vi "GUI control.vi"() -> ()   [LabVIEW 2018]
doc: "This example performs a serial port write and a serial port read. The parameters set for the serial port must match the parameters of the connected instrument or device. The VISA Configure Serial Port VI sets the configuration parameters. The front panel displays the controls used to configure the basic parameters, such as baud rate, data bits, and parity. The VI passes the VISA resource name to other VIs that perform operations on that VISA resource. The VISA Write function sends a command to the serial device and the VISA Read function returns data based on the command. The VISA Close function then closes the reference to the serial device. It is important to close the reference; otherwise, further communication through that port might not be possible."
uses:
  Program Files/National Instruments/LabVIEW 2018/examples/Instrument IO/Serial/support/Serial - Settings.ctl
  <vilib>/Instr/_visa.llb/VISA Configure Serial Port (Instr).vi
  <vilib>/Utility/file.llb/Write Delimited Spreadsheet (string).vi
panel:
  in  "file path 1D":path
  in  "file path static":path
  out "Magnetic field z [µT]":dbl
  out "Magnetic field y [µT]":dbl
  out "Magnetic field x [µT]":dbl
  out "Magnetic field strength [µT]":dbl
  in  "Direction field sweep":string(combo)
  in  "Minimum value B [µT]":dbl
  in  "Maximum value B [µT]":dbl
  in  "START":bool
  in  "Number of steps":dbl
  out "Current has stabilized":bool
  in  "Next iteration 2":bool
  in  "Starting step":dbl
  out "Current has stabilized":bool
  out "Current has stabilized":bool
  in  "Next iteration":bool
  in  "file path 3D":path
  in  "Start":bool
  out "Start time 2":timestamp
  out "Angle \"phi\"":dbl
  out "Current iteration":i32
  in  "Number of steps":dbl
  in  "Angle theta [degrees]":dbl
  in  "Magnetic field strength [µT]":dbl
  in  "Octant":string(combo)
  in  "Sweep plane & fixed axis":string(combo)
  in  "OFF":bool
  in  "OK Button":bool
  in  "Magnetic field strength z [µT]":dbl
  in  "Magnetic field strength y [µT]":dbl
  in  "Magnetic field strength x [µT]":dbl
  in  "Static or field sweep?":string(combo)
  in  "Serial Settings":T1={"baud rate"=9600, "data bits"=8, "parity"=enum."None", "stop bits"=10, "flow control"=0} {"flow control" items=["None"=0, "XON/XOFF"=1, "RTS/CTS"=2, "DTR/DSR"=4]; "stop bits" items=["1.0"=10, "1.5"=15, "2.0"=20]; "data bits" min=5 max=8 step=1; "baud rate" items=["75"=75, "110"=110, "134"=134, "150"=150, "300"=300, "600"=600, "1200"=1200, "1800"=1800, "2400"=2400, "4800"=4800, "7200"=7200, "9600"=9600, "14400"=14400, "19200"=19200, "28800"=28800, "38400"=38400, "56000"=56000, "57600"=57600, "115200"=115200, "128000"=128000, "230400"=230400]}
  in  "VISA resource name":refnum<visa-resource-name>="COM1"
  # "Static field"
  # "1D magnitude sweep"
  # "Settings"
  # "3D field sweep"
  # "About the 3D field sweep"
  # "A onstant-magnitude, fixed-tilt, azimuthal sweep of a 3D vector is performed.\nThe mag,netic field vector is angled away from a fixed axis by a certain angle \"phi\". It then makes a circular motion around that fixed axis, eventually tracing out a full cone.\nYou choose a plane of variation ( x–y, x–z, or y–z) and hold one direction constant (e.g., z).  The sweep is performed clockwise, as seen from the origin."
  # "File paths must be a csv comma delimited excell file!"
  # "How to connect the cables"
  # "Current state"
  # "Current state"
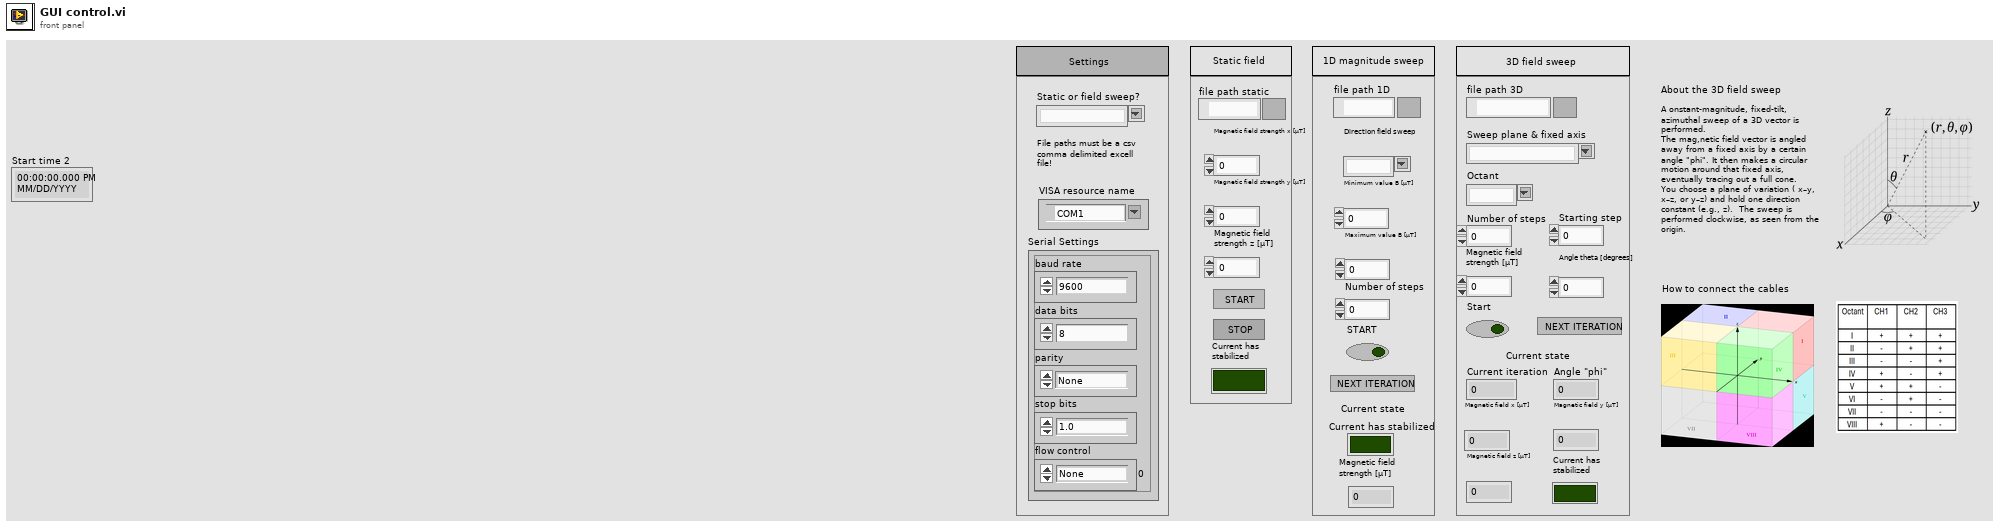
[diagram p1: front panel]
types:
  T1 = typedef "Serial - Settings.ctl" = cluster{"baud rate":u32, "data bits":u16, "parity":enum16{"None", "Odd", "Even", "Mark", "Space"}, "stop bits":u16, "flow control":u16}
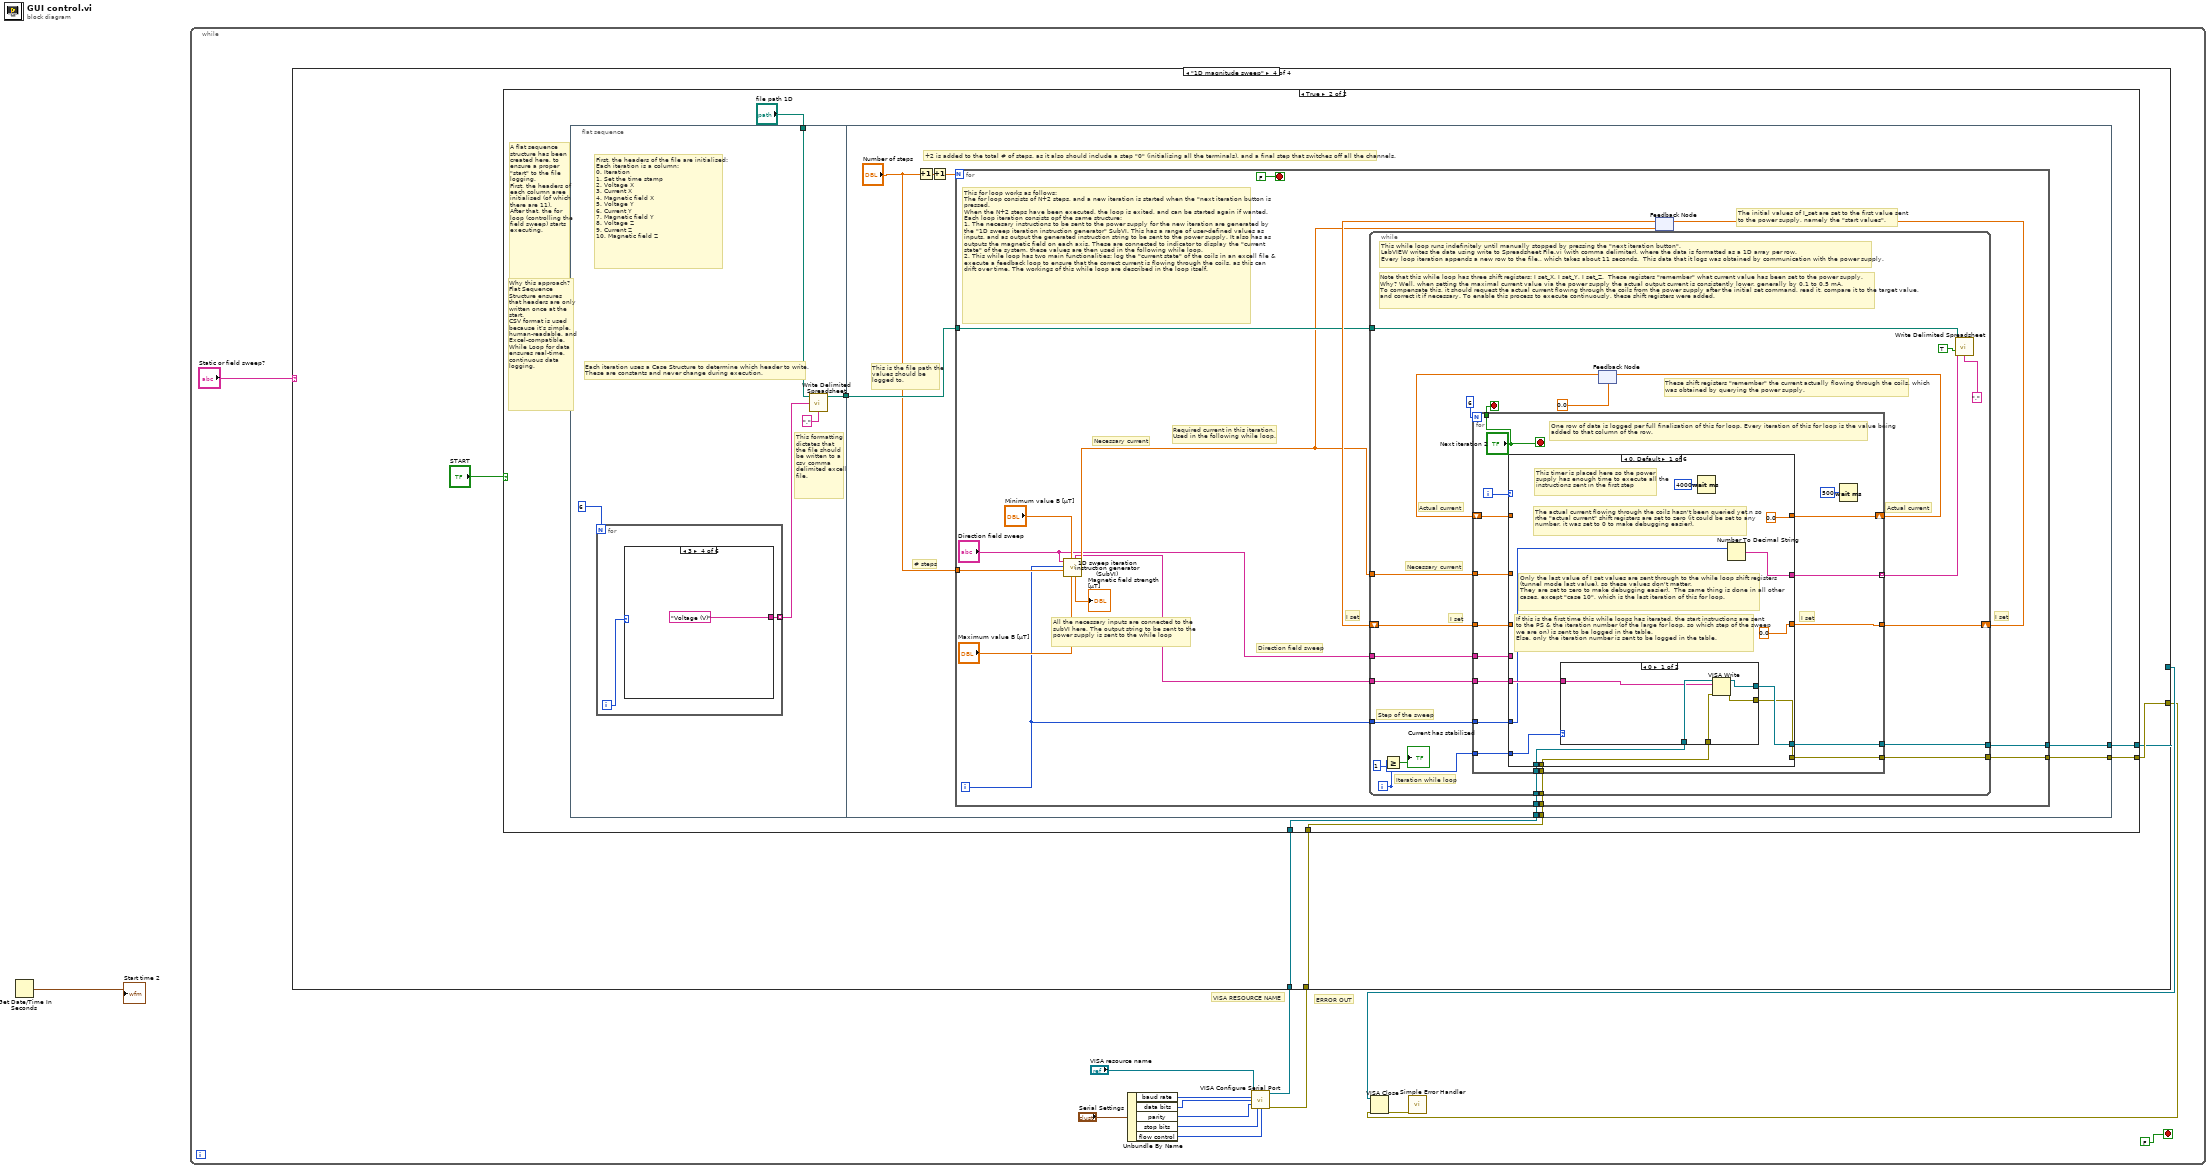
[diagram p0: block diagram]
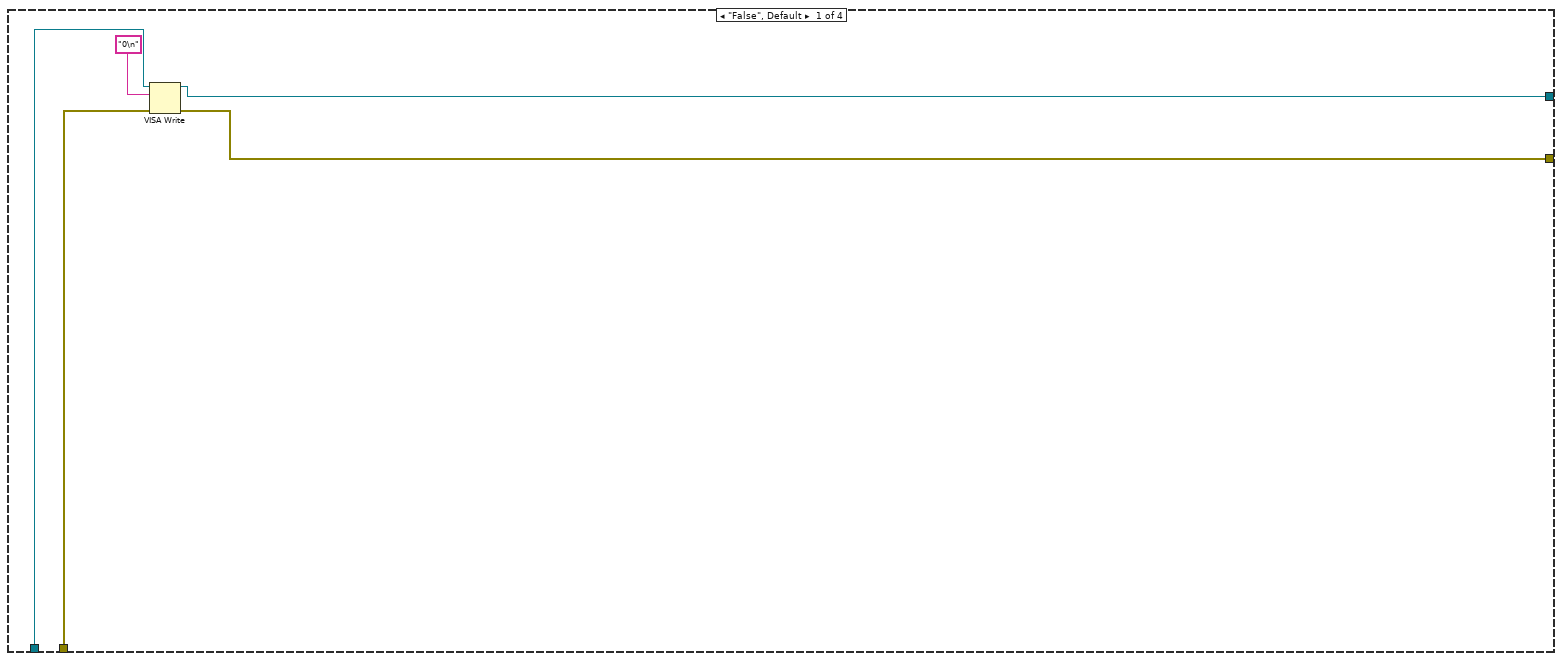
[diagram p2: hidden frame]
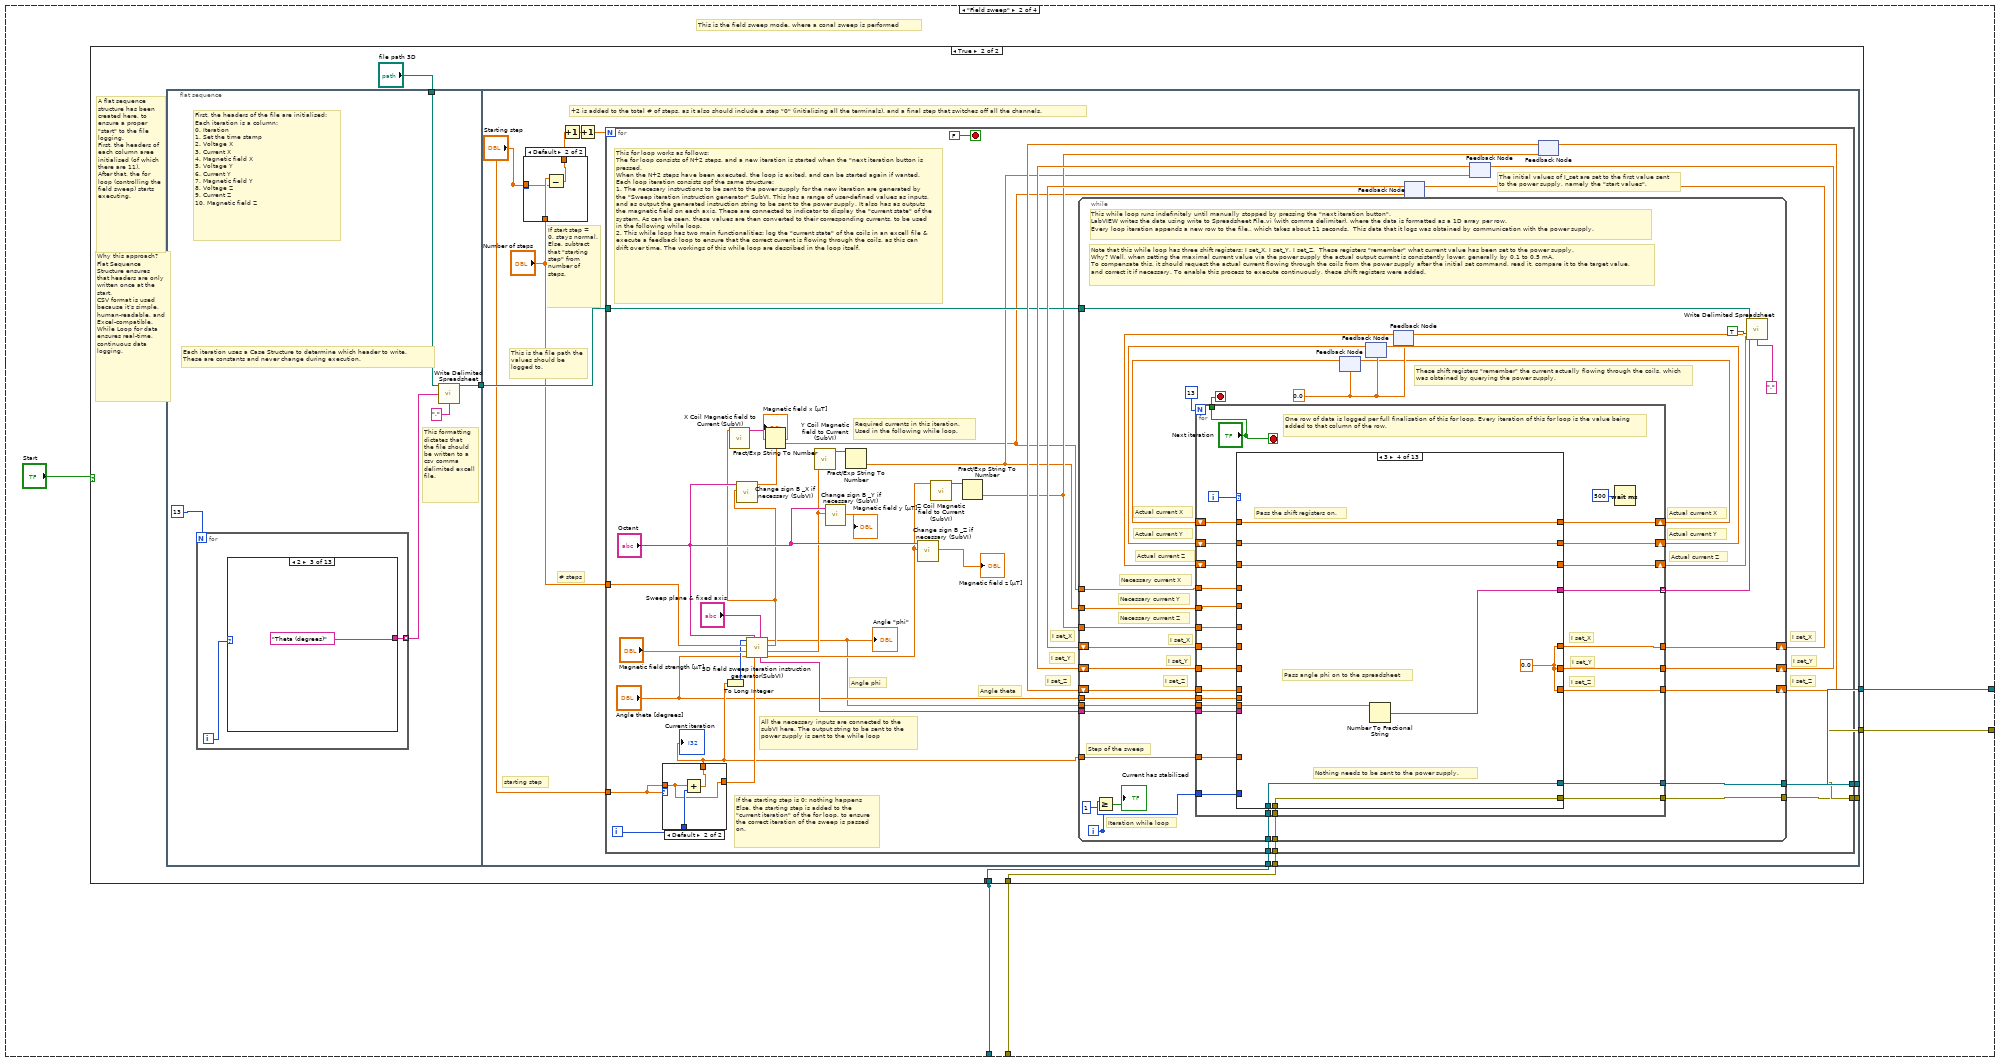
[diagram p3: hidden frame]
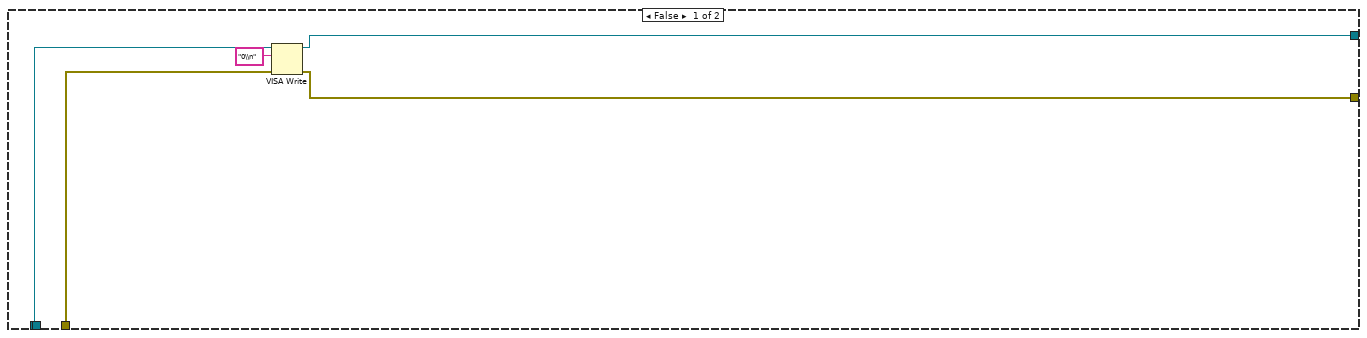
[diagram p4: hidden frame]
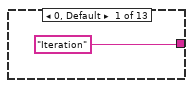
[diagram p5: hidden frame]
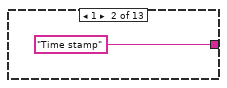
[diagram p6: hidden frame]
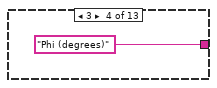
[diagram p7: hidden frame]
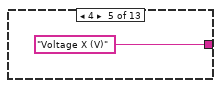
[diagram p8: hidden frame]
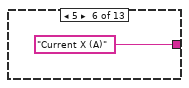
[diagram p9: hidden frame]
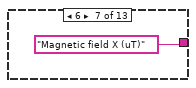
[diagram p10: hidden frame]
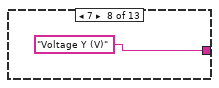
[diagram p11: hidden frame]
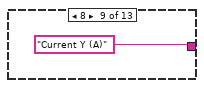
[diagram p12: hidden frame]
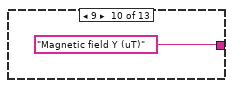
[diagram p13: hidden frame]
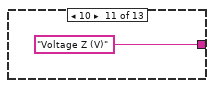
[diagram p14: hidden frame]
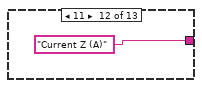
[diagram p15: hidden frame]
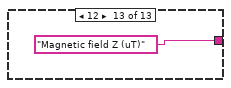
[diagram p16: hidden frame]
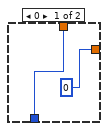
[diagram p18: hidden frame]
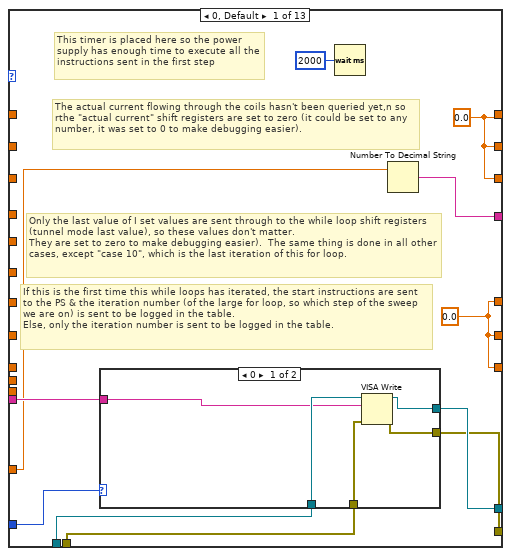
[diagram p19: hidden frame]
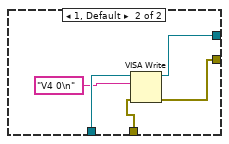
[diagram p20: hidden frame]
diagram:
  n1 = Get Date/Time In Seconds() -> (seconds since 1Jan1904=→"Start time 2":timestamp)
  n2 = while {
    stop <- FALSE stop-if-true
    # "VISA RESOURCE NAME"
    # "ERROR OUT"
    n3 = Unbundle By Name("Serial Settings") -> ("baud rate"=w12:u32, "data bits"=w2:u16, "parity"=w11:enum16{"None", "Odd", "Even", "Mark", "Space"}, "stop bits"=w10:u16, "flow control"=w9:u16)
    n4 = call-poly "VISA Configure Serial Port"("VISA resource name"="VISA resource name", "baud rate (9600)"=w12, "data bits (8)"=w2, "parity (0:none)"=w11, "stop bits (10: 1 bit)"=w10, "flow control (0:none)"=w9) -> ("VISA resource name out"=w3:refnum<visa-resource-name>, "error out"=w8:errorcluster)  [unwired: 3 in, 5 out]
    n5 = case shown="\"1D magnitude sweep\"" "Static or field sweep?" {
      tunnel: [w16 w24 w444 w813] -> w6
      tunnel: w3 -> [w18 w22 w441 w815]
      tunnel: w8 -> [w19 w23 w445 w814]
      tunnel: [w17 w25 w443 w812] -> w7
      frame "False", Default {
        n6 = VISA Write(VISA resource name=w18, write buffer="0\n", error in (no error)=w19) -> (VISA resource name out=w17:refnum<visa-resource-name>, error out=w16:errorcluster)  [unwired: 1 out]
      }
      frame "Field sweep" {
        # "This is the field sweep mode, where a conal sweep is performed"
        n7 = case shown="True" "Start" {
          tunnel: [w30 w34] -> w25
          tunnel: [w29 w33] -> w24
          tunnel: w22 -> [w27 w36]
          tunnel: w23 -> [w28 w35]
          tunnel: w22 -> [_ _]
          frame False {
            n8 = VISA Write(VISA resource name=w27, write buffer="0\\n", error in (no error)=w28) -> (VISA resource name out=w30:refnum<visa-resource-name>, error out=w29:errorcluster)  [unwired: 1 out]
          }
          frame True {
            # "Why this approach?\nFlat Sequence Structure ensures that headers are only written once at the start.\nCSV format is used because it’s simple, human-readable, and Excel-compatible.\nWhile Loop for data ensures real-time, continuous data logging."
            # "A flat sequence structure has been created here, to ensure a proper \"start\" to the file logging. \nFirst, the headers of each column aree initialised (of which there are 11). \nAfter that, the for loop (controlling the field sweep) starts executing."
            n9 = flat-sequence {
              tunnel: "file path 3D" -> [w38]
              tunnel: [w37] -> w32
              tunnel: w36 -> [w64]
              tunnel: w35 -> [w63]
              tunnel: [w62] -> w34
              tunnel: [w61] -> w33
              tunnel: w32 -> [w60]
              frame #0 {
                # "Each iteration uses a Case Structure to determine which header to write.\nThese are constants and never change during execution."
                # "This formatting dictates that the file should be written to a csv comma delimited excell file."
                # "First, the headers of the file are initialised:\nEach iteration is a column:\n0. Iteration\n1. Set the time stamp\n2. Voltage X\n3. Current X\n4. Magnetic field X\n5. Voltage Y\n6. Current Y\n7. Magnetic field Y\n8. Voltage Z\n9. Current Z\n10. Magnetic field Z"
                n10 = for {
                  N: 13 -> [_]
                  tunnel: [w42] -> w40 mode=indexing
                  i -> [w43]
                  n11 = case shown="2" w43 {
                    tunnel: ["Iteration" "Time stamp" "Theta (degrees)" "Phi (degrees)" "Voltage X (V)" "Current X (A)" "Magnetic field X (uT)" "Voltage Y (V)" "Current Y (A)" "Magnetic field Y (uT)" "Voltage Z (V)" "Current Z (A)" "Magnetic field Z (uT)"] -> w42
                    frame 0, Default {
                    }
                    frame 1 {
                    }
                    frame 2 {
                    }
                    frame 3 {
                    }
                    frame 4 {
                    }
                    frame 5 {
                    }
                    frame 6 {
                    }
                    frame 7 {
                    }
                    frame 8 {
                    }
                    frame 9 {
                    }
                    frame 10 {
                    }
                    frame 11 {
                    }
                    frame 12 {
                    }
                  }
                }
                n12 = call-poly <vilib>:"Write Delimited Spreadsheet.vi"("file path (dialog if empty)"=w38, "1D data"=w40, "delimiter (\\t)"="," ("delimiter (\\t)")) -> ("new file path (Not A Path if cancelled)"=w37:path)  [unwired: 11 in, 1 out]
              }
              frame #1 {
                # "starting step"
                # "# steps"
                # "If start step = 0, stays normal.\nElse, subtract that \"starting step\" from number of steps."
                # "This is the file path the values should be logged to."
                # "+2 is added to the total # of steps, as it also should include a step \"0\" (initialising all the terminals), and a final step that switches off all the channels."
                n13 = case shown="Default" "Starting step" {
                  tunnel: "Number of steps" -> [w67 w70]
                  tunnel: [w67 w69] -> w58
                  tunnel: "Starting step" -> [_ w68]
                  frame 0 {
                  }
                  frame Default {
                    n14 = Subtract(x=w70, y=w68) -> (x-y=w69:dbl)
                  }
                }
                n15 = Increment(x=w58) -> (x+1=w66:dbl)
                n16 = Increment(x=w66) -> (x+1=w65:dbl)
                n17 = for {
                  N: w65 -> [_]
                  tunnel: "Number of steps" -> [w101]
                  tunnel: w64 -> [w92]
                  tunnel: w63 -> [w91]
                  tunnel: [w90] -> w62
                  tunnel: [w89] -> w61
                  tunnel: w60 -> [w88]
                  tunnel: "Starting step" -> [w80]
                  i -> [w81]
                  stop <- FALSE stop-if-true
                  # "Angle phi"
                  # "Angle theta"
                  # "If the starting step is 0: nothing happens\nElse, the starting step is added to the \"current iteration\" of the for loop, to ensure the correct iteration of the sweep is passed on."
                  # "The initial values of I_set are set to the first value sent to the power supply, namely the \"start values\"."
                  # "All the necessary inputs are connected to the subVI here. The output string to be sent to the power supply is sent to the while loop"
                  # "This for loop works as follows: \nThe for loop consists of N+2 steps, and a new iteration is started when the \"next iteration button is pressed.\nWhen the N+2 steps have been executed, the loop is exited, and can be started again if wanted.\nEach loop iteration consists opf the same structure:\n1. The necesary instructions to be sent to the power supply for the new iteration are generated by the \"Sweep iteration instruction generator\" SubVI. This has a range of user-defined values as inputs, and as output the generated instruction string to be sent to the power supply. It also has as outputs the magnetic field on each axis. These are connected to indicator to display the \"current state\" of the system. As can be seen, these values are then converted to their corresponding currents, to be used in the following while loop.\n2. This while loop has two main functionalities: log the \"current state\" of the coils in an excell file & execute a feedback loop to ensure that the correct current is flowing through the coils, as this can drift over time. The workings of this while loop are described in the loop itself."
                  # "I set_Z"
                  # "I set_Y"
                  # "I set_Y"
                  # "I set_Z"
                  # "I set_X"
                  # "I set_X"
                  # "Required currents in this iteration. \nUsed in the following while loop."
                  n18 = case shown="Default" w80 {
                    tunnel: w81 -> [w108 w111]
                    tunnel: [w108 w110] -> w75
                    tunnel: w80 -> [_ w109]
                    tunnel: [0 ("y") w109] -> w79
                    frame 0 {
                    }
                    frame Default {
                      n19 = Add(x=w109, y=w111) -> (x+y=w110:dbl)
                    }
                  }
                  "Current iteration" <- w75
                  n20 = To Long Integer(number=w75) -> (32bit integer=w74:i32)
                  n21 = call "3D field sweep iteration instruction generator(SubVI).vi"("Sweep plane & fixed axis"="Sweep plane & fixed axis", "Sweep starts later"=w79, "Octant"="Octant", "Angle theta [degrees]"="Angle theta [degrees]", "Magnetic field strength [µT]"="Magnetic field strength [µT]", "Number of steps"=w101, "Current iteration"=w74) -> ("Magnetic field z [µT]"=w76:dbl, "Magnetic field y [µT]"=w77:dbl, "Magnetic field x [µT]"=w78:dbl, "Azimuthal angle \"phi\""=w71:dbl, "Output string instruction"=w93:string)
                  "Angle \"phi\"" <- w71
                  n22 = call "X Coil Magnetic field to Current (SubVI).vi"("Magnetic field [µT]"=w78) -> ("Current X"=w103:string)  [unwired: 10 in]
                  n23 = call "Change sign B _X if necessary (SubVI).vi"("Magnetic field x [µT] in"=w78, "Octant"="Octant") -> ("Magnetic field x [µT] out"=→"Magnetic field x [µT]":dbl)  [unwired: 9 in]
                  n24 = Fract/Exp String To Number(string=w103) -> (number=w82:dbl)  [unwired: 3 in, 1 out]
                  n25 = call "Y Coil Magnetic field to Current (SubVI).vi"("Magnetic field [µT]"=w77) -> ("Current Y"=w104:string)  [unwired: 10 in]
                  n26 = call "Change sign B _Y if necessary (SubVI).vi"("Magnetic field y [µT]  in"=w77, "Octant"="Octant") -> ("Magnetic field y [µT]  out"=→"Magnetic field y [µT]":dbl)  [unwired: 9 in]
                  n27 = Fract/Exp String To Number(string=w104) -> (number=w86:dbl)  [unwired: 3 in, 1 out]
                  n28 = call "Change sign B _Z if necessary (SubVI).vi"("Magnetic field z [µT] in"=w76, "Octant"="Octant") -> ("Magnetic field z [µT] out"=→"Magnetic field z [µT]":dbl)  [unwired: 9 in]
                  n29 = call "Z Coil Magnetic field to Current (SubVI).vi"("Magnetic field [µT]"=w76) -> ("Current Z"=w105:string)  [unwired: 10 in]
                  n30 = Fract/Exp String To Number(string=w105) -> (number=w87:dbl)  [unwired: 3 in, 1 out]
                  n31 = feedback #1(w82) -> (w99:dbl)
                  n32 = feedback #2(w86) -> (w96:dbl)
                  n33 = feedback #3(w87) -> (w94:dbl)
                  n34 = while {
                    tunnel: w88 -> [w141]
                    tunnel: w92 -> [w138]
                    tunnel: w91 -> [w137]
                    tunnel: [w136] -> w89
                    tunnel: [w135] -> w90
                    tunnel: w75 -> [w128]
                    shift-right: [w127] -> w98
                    shift-left: w99 -> [w126]
                    tunnel: w93 -> [w125]
                    shift-right: [w124] -> w97
                    shift-left: w96 -> [w122]
                    shift-right: [w123] -> w95
                    shift-left: w94 -> [w121]
                    tunnel: w82 -> [w120]
                    tunnel: w86 -> [w119]
                    tunnel: w87 -> [w118]
                    tunnel: "Angle theta [degrees]" -> [w113]
                    tunnel: w71 -> [w112]
                    i -> [w117]
                    stop <- w114 stop-if-true
                    w130 = 0.0
                    # "These shift registers \"remember\" the current actually flowing through the coils, which was obtained by querying the power supply."
                    # "Note that this while loop has three shift registers: I set_X, I set_Y, I set_Z.  These registers \"remember\" what current value has been set to the power supply. \nWhy? Well, when setting the maximal current value via the power supply the actual output current is consistently lower, generally by 0.1 to 0.5 mA.\nTo compensate this, it should request the actual current flowing through the coils from the power supply after the initial set command, read it, compare it to the target value, and correct it if necessary. To enable this process to execute continuously, these shift registers were added."
                    # "This while loop runs indefinitely until manually stopped by pressing the \"next iteration button\". \nLabVIEW writes the data using write to Spreadsheet File.vi (with comma delimiter), where the data is formatted as a 1D array per row.\nEvery loop iteration appends a new row to the file,, which takes about 11 seconds.  This data that it logs was obtained by communication with the power supply."
                    # "Necessary current Z"
                    # "Necessary current Y"
                    # "Necessary current X"
                    # "I set_Z"
                    # "I set_Y"
                    # "Iteration while loop"
                    # "Step of the sweep"
                    # "I set_X"
                    # "Actual current Z"
                    # "Actual current Y"
                    # "Actual current X"
                    # "Actual current Z"
                    # "Actual current Y"
                    # "Actual current X"
                    n35 = Greater Or Equal?(x=w117, y=1) -> (x >= y?=→"Current has stabilized":bool)
                    n36 = feedback #4(w130) -> (w143:dbl)
                    n37 = feedback #5(w130) -> (w133:dbl)
                    n38 = feedback #6(w130) -> (w131:dbl)
                    n39 = for {
                      N: 13 -> [_]
                      tunnel: [w170] -> w142 mode=indexing
                      shift-right: [w165] -> w129
                      shift-left: w143 -> [w172]
                      tunnel: w138 -> [w169]
                      tunnel: w137 -> [w168]
                      tunnel: [w167] -> w136
                      tunnel: [w166] -> w135
                      shift-right: [w162] -> w134
                      shift-left: w133 -> [w164]
                      shift-right: [w161] -> w132
                      shift-left: w131 -> [w163]
                      tunnel: w117 -> [w160]
                      tunnel: w128 -> [w159]
                      tunnel: w126 -> [w158]
                      tunnel: [w157] -> w127
                      tunnel: w125 -> [w156]
                      tunnel: [w155] -> w124
                      tunnel: [w154] -> w123
                      tunnel: w122 -> [w153]
                      tunnel: w121 -> [w152]
                      tunnel: w120 -> [w151]
                      tunnel: w119 -> [w150]
                      tunnel: w118 -> [w149]
                      tunnel: ["Next iteration"] -> w114
                      tunnel: w113 -> [w146]
                      tunnel: w112 -> [w145]
                      i -> [w171]
                      stop <- "Next iteration" stop-if-true
                      # "One row of data is logged per full finalisation of this for loop. Every iteration of this for loop is the value being added to that column of the row."
                      # "I set_Y"
                      # "I set_Z"
                      # "I set_X"
                      n40 = case shown="3" w171 {
                        tunnel: [w177 w200 w209 w213 w220 w247 w269 w279 w298 w321 w333 w356 w393] -> w170
                        tunnel: w169 -> [w180 w199 w204 w212 w235 w256 w271 w281 w305 w325 w335 w360 w386]
                        tunnel: w168 -> [w181 w198 w203 w211 w234 w257 w270 w280 w306 w326 w334 w359 w385]
                        tunnel: [w183 w199 w204 w212 w233 w259 w271 w275 w303 w325 w332 w358 w388] -> w166
                        tunnel: [w182 w198 w203 w211 w232 w258 w270 w274 w302 w326 w331 w357 w387] -> w167
                        tunnel: [w179 w197 w208 w217 w239 w248 w272 w278 w300 w324 w330 w355 w392] -> w165
                        tunnel: w172 -> [_ w197 w208 w217 w239 _ w272 w278 w300 w324 w330 w355 w392]
                        tunnel: w164 -> [_ w196 w207 w216 w223 w245 w268 w277 _ w322 w329 w354 w384]
                        tunnel: w163 -> [_ w195 w206 w215 w222 w244 w267 w276 w299 w323 w328 _ w380]
                        tunnel: [w179 w196 w207 w216 w223 w245 w268 w277 w301 w322 w329 w354 w384] -> w162
                        tunnel: [w179 w195 w206 w215 w222 w244 w267 w276 w299 w323 w328 w353 w380] -> w161
                        tunnel: w160 -> [w178 _ _ _ _ _ _ _ _ _ _ _ w375]
                        tunnel: w159 -> [w174 _ _ _ _ _ _ _ _ _ _ _ _]
                        tunnel: [w175 w194 w205 w218 w219 w243 w266 w273 w297 w320 w327 w352 w389] -> w157
                        tunnel: w158 -> [_ _ _ _ _ _ _ _ _ _ _ _ w391]
                        tunnel: w156 -> [w176 _ _ _ _ _ _ _ _ _ _ _ _]
                        tunnel: [w175 w194 w205 w218 w219 w243 w266 w273 w297 w320 w327 w352 w381] -> w155
                        tunnel: [w175 w194 w205 w218 w219 w243 w266 w273 w297 w320 w327 w352 w377] -> w154
                        tunnel: w153 -> [_ _ _ _ _ _ _ _ _ _ _ _ w383]
                        tunnel: w152 -> [_ _ _ _ _ _ _ _ _ _ _ _ w378]
                        tunnel: w151 -> [_ _ _ _ _ _ _ _ _ _ _ _ w390]
                        tunnel: w150 -> [_ _ _ _ _ _ _ _ _ _ _ _ w382]
                        tunnel: w149 -> [_ _ _ _ _ _ _ _ _ _ _ _ w379]
                        tunnel: w146 -> [_ _ w210 _ _ _ _ _ _ _ _ _ _]
                        tunnel: w145 -> [_ _ _ w214 _ _ _ _ _ _ _ _ _]
                        frame 0, Default {
                          w175 = 0.0
                          w179 = 0.0
                          # "This timer is placed here so the power supply has enough time to execute all the instructions sent in the first step"
                          # "Only the last value of I set values are sent through to the while loop shift registers (tunnel mode last value), so these values don't matter. \nThey are set to zero to make debugging easier).  The same thing is done in all other cases, except \"case 10\", which is the last iteration of this for loop."
                          # "The actual current flowing through the coils hasn't been queried yet,n so rthe \"actual current\" shift registers are set to zero (it could be set to any number, it was set to 0 to make debugging easier)."
                          # "If this is the first time this while loops has iterated, the start instructions are sent to the PS & the iteration number (of the large for loop, so which step of the sweep we are on) is sent to be logged in the table.\nElse, only the iteration number is sent to be logged in the table."
                          n41 = case shown="0" w178 {
                            tunnel: [w188 w193] -> w183
                            tunnel: [w187 w192] -> w182
                            tunnel: w181 -> [w186 w191]
                            tunnel: w180 -> [w185 w190]
                            tunnel: w176 -> [w184 _]
                            frame 0 {
                              n42 = VISA Write(VISA resource name=w185, write buffer=w184, error in (no error)=w186) -> (VISA resource name out=w188:refnum<visa-resource-name>, error out=w187:errorcluster)  [unwired: 1 out]
                            }
                            frame 1, Default {
                              n43 = VISA Write(VISA resource name=w190, write buffer="V4 0\n", error in (no error)=w191) -> (VISA resource name out=w193:refnum<visa-resource-name>, error out=w192:errorcluster)  [unwired: 1 out]
                            }
                          }
                          n44 = Wait (ms)(milliseconds to wait=u32 2000) -> ()  [unwired: 1 out]
                          n45 = Number To Decimal String(number=w174) -> (decimal integer string=w177:string)  [unwired: 1 in]
                        }
                        frame 1 {
                          w194 = 0.0
                          # "Nothing needs to be sent to the power supply."
                          # "Pass the shift registers on."
                          # "only send the time, not the date"
                          # "Send the time stamp to be logged"
                          n46 = Get Date/Time In Seconds() -> (seconds since 1Jan1904=w202:timestamp)
                          n47 = Format Date/Time String(time format string (%c)="%H:%M:%S", seconds (now)=w202) -> (date/time string=w200:string)  [unwired: 1 in]
                        }
                        frame 2 {
                          w205 = 0.0
                          # "Nothing needs to be sent to the power supply."
                          # "Pass the shift registers on."
                          # "Pass angle theta to the spreadsheet"
                          n48 = Number To Fractional String(number=w210) -> (F-format string=w209:string)  [unwired: 3 in]
                        }
                        frame 3 {
                          w218 = 0.0
                          # "Nothing needs to be sent to the power supply."
                          # "Pass angle phi on to the spreadsheet"
                          # "Pass the shift registers on."
                          n49 = Number To Fractional String(number=w214) -> (F-format string=w213:string)  [unwired: 3 in]
                        }
                        frame 4 {
                          w219 = 0.0
                          # "Pass the shift registers on."
                          # "The answer back from the PS is in the form x V. This V needs to be removed, otherwise the table formats wrong."
                          # "Request voltage CH1 & write it to the file"
                          n50 = call "Request voltage CH1 (SubVI).vi"() -> ("Request voltage CH1 / X"=w225:string)  [unwired: 11 in]
                          n51 = VISA Write(VISA resource name=w235, write buffer=w225, error in (no error)=w234) -> (VISA resource name out=w238:refnum<visa-resource-name>, error out=w237:errorcluster)  [unwired: 1 out]
                          n52 = flat-sequence {
                            tunnel: w237 -> [w240]
                            tunnel: w238 -> [w241]
                            tunnel: [w241] -> w231
                            tunnel: u32 500 ("delay before read (ms) static") -> [w242]
                            tunnel: [w240] -> w230
                            frame #0 {
                              n53 = Wait (ms)(milliseconds to wait=w242) -> ()  [unwired: 1 out]
                            }
                          }
                          n54 = property class="Instr"(reference=w231, error in=w230) -> (reference out=w229:refnum<visa-resource-name>, error out=w228:errorcluster, "Serial Settings:Number of Bytes at Serial Port"=w227:u32)
                          n55 = VISA Read(VISA resource name=w229, byte count=w227, error in (no error)=w228) -> (VISA resource name out=w233:refnum<visa-resource-name>, read buffer=w224:string, error out=w232:errorcluster)  [unwired: 1 out]
                          n56 = Scan From String(format string="%fV", input string=w224) -> (output 1=w221:dbl)  [unwired: 3 in, 3 out]
                          n57 = Number To Fractional String(number=w221) -> (F-format string=w220:string)  [unwired: 3 in]
                        }
                        frame 5 {
                          w243 = 0.0
                          # "Pass the shift registers on."
                          # "The answer back from the PS is in the form x A. This A needs to be removed, otherwise the table formats wrong."
                          # "Request current CH1; write it to the file; put it on the current X shift register"
                          n58 = call "Request current CH1(SubVI).vi"() -> ("Request current CH1 / X"=w249:string)  [unwired: 11 in]
                          n59 = VISA Write(VISA resource name=w256, write buffer=w249, error in (no error)=w257) -> (VISA resource name out=w262:refnum<visa-resource-name>, error out=w261:errorcluster)  [unwired: 1 out]
                          n60 = flat-sequence {
                            tunnel: w261 -> [w263]
                            tunnel: w262 -> [w264]
                            tunnel: [w264] -> w254
                            tunnel: u32 500 ("delay before read (ms) static") -> [w265]
                            tunnel: [w263] -> w253
                            frame #0 {
                              n61 = Wait (ms)(milliseconds to wait=w265) -> ()  [unwired: 1 out]
                            }
                          }
                          n62 = property class="Instr"(reference=w254, error in=w253) -> (reference out=w252:refnum<visa-resource-name>, error out=w250:errorcluster, "Serial Settings:Number of Bytes at Serial Port"=w251:u32)
                          n63 = VISA Read(VISA resource name=w252, byte count=w251, error in (no error)=w250) -> (VISA resource name out=w259:refnum<visa-resource-name>, read buffer=w255:string, error out=w258:errorcluster)  [unwired: 1 out]
                          n64 = Scan From String(format string="%fA", input string=w255) -> (output 1=w248:dbl)  [unwired: 3 in, 3 out]
                          n65 = Number To Fractional String(number=w248) -> (F-format string=w247:string)  [unwired: 3 in]
                        }
                        frame 6 {
                          w266 = 0.0
                          # "Pass the shift registers on."
                          # "Send magnetic field X to log file"
                          n66 = call "X Coil Current to Magnetic field (SubVI).vi"("Current X"=w272) -> ("Magnetic field X [µT]"=w269:string)  [unwired: 10 in]
                        }
                        frame 7 {
                          w273 = 0.0
                          # "Pass the shift registers on."
                          # "The answer back from the PS is in the form x V. This V needs to be removed, otherwise the table formats wrong."
                          # "Request voltage CH2 & write it to the file"
                          n67 = call "Request voltage CH2 (SubVI).vi"() -> ("Request voltage CH2 / Y"=w282:string)  [unwired: 11 in]
                          n68 = VISA Write(VISA resource name=w281, write buffer=w282, error in (no error)=w280) -> (VISA resource name out=w293:refnum<visa-resource-name>, error out=w292:errorcluster)  [unwired: 1 out]
                          n69 = flat-sequence {
                            tunnel: w292 -> [w294]
                            tunnel: w293 -> [w295]
                            tunnel: [w295] -> w290
                            tunnel: u32 500 ("delay before read (ms) static") -> [w296]
                            tunnel: [w294] -> w289
                            frame #0 {
                              n70 = Wait (ms)(milliseconds to wait=w296) -> ()  [unwired: 1 out]
                            }
                          }
                          n71 = property class="Instr"(reference=w290, error in=w289) -> (reference out=w288:refnum<visa-resource-name>, error out=w287:errorcluster, "Serial Settings:Number of Bytes at Serial Port"=w286:u32)
                          n72 = VISA Read(VISA resource name=w288, byte count=w286, error in (no error)=w287) -> (VISA resource name out=w275:refnum<visa-resource-name>, read buffer=w284:string, error out=w274:errorcluster)  [unwired: 1 out]
                          n73 = Scan From String(format string="%fV", input string=w284) -> (output 1=w283:dbl)  [unwired: 3 in, 3 out]
                          n74 = Number To Fractional String(number=w283) -> (F-format string=w279:string)  [unwired: 3 in]
                        }
                        frame 8 {
                          w297 = 0.0
                          # "Pass the shift registers on."
                          # "The answer back from the PS is in the form x A. This A needs to be removed, otherwise the table formats wrong."
                          # "Request current CH2; write it to the file; put it on the current Y shift register"
                          n75 = call "Request current CH2 (SubVI).vi"() -> ("Request current CH2 / Y"=w304:string)  [unwired: 11 in]
                          n76 = VISA Write(VISA resource name=w305, write buffer=w304, error in (no error)=w306) -> (VISA resource name out=w316:refnum<visa-resource-name>, error out=w315:errorcluster)  [unwired: 1 out]
                          n77 = flat-sequence {
                            tunnel: w315 -> [w317]
                            tunnel: w316 -> [w318]
                            tunnel: [w318] -> w312
                            tunnel: u32 500 ("delay before read (ms) static") -> [w319]
                            tunnel: [w317] -> w311
                            frame #0 {
                              n78 = Wait (ms)(milliseconds to wait=w319) -> ()  [unwired: 1 out]
                            }
                          }
                          n79 = property class="Instr"(reference=w312, error in=w311) -> (reference out=w310:refnum<visa-resource-name>, error out=w308:errorcluster, "Serial Settings:Number of Bytes at Serial Port"=w309:u32)
                          n80 = VISA Read(VISA resource name=w310, byte count=w309, error in (no error)=w308) -> (VISA resource name out=w303:refnum<visa-resource-name>, read buffer=w313:string, error out=w302:errorcluster)  [unwired: 1 out]
                          n81 = Scan From String(format string="%fA", input string=w313) -> (output 1=w301:dbl)  [unwired: 3 in, 3 out]
                          n82 = Number To Fractional String(number=w301) -> (F-format string=w298:string)  [unwired: 3 in]
                        }
                        frame 9 {
                          w320 = 0.0
                          # "Pass the shift registers on."
                          # "Send magnetic field Y to log file"
                          n83 = call "Y Coil Current to Magnetic field (SubVI).vi"("Current Y"=w322) -> ("Magnetic field Y [µT]"=w321:string)  [unwired: 10 in]
                        }
                        frame 10 {
                          w327 = 0.0
                          # "Pass the shift registers on."
                          # "The answer back from the PS is in the form x V. This V needs to be removed, otherwise the table formats wrong."
                          # "Request voltage CH3 & write it to the file"
                          n84 = call "Request voltage CH3 (SubVI).vi"() -> ("Request voltage CH3 / Z"=w336:string)  [unwired: 11 in]
                          n85 = VISA Write(VISA resource name=w335, write buffer=w336, error in (no error)=w334) -> (VISA resource name out=w347:refnum<visa-resource-name>, error out=w346:errorcluster)  [unwired: 1 out]
                          n86 = flat-sequence {
                            tunnel: w346 -> [w348]
                            tunnel: w347 -> [w349]
                            tunnel: [w349] -> w344
                            tunnel: u32 500 ("delay before read (ms) static") -> [w350]
                            tunnel: [w348] -> w343
                            frame #0 {
                              n87 = Wait (ms)(milliseconds to wait=w350) -> ()  [unwired: 1 out]
                            }
                          }
                          n88 = property class="Instr"(reference=w344, error in=w343) -> (reference out=w342:refnum<visa-resource-name>, error out=w341:errorcluster, "Serial Settings:Number of Bytes at Serial Port"=w340:u32)
                          n89 = VISA Read(VISA resource name=w342, byte count=w340, error in (no error)=w341) -> (VISA resource name out=w332:refnum<visa-resource-name>, read buffer=w338:string, error out=w331:errorcluster)  [unwired: 1 out]
                          n90 = Scan From String(format string="%fV", input string=w338) -> (output 1=w337:dbl)  [unwired: 3 in, 3 out]
                          n91 = Number To Fractional String(number=w337) -> (F-format string=w333:string)  [unwired: 3 in]
                        }
                        frame 11 {
                          w352 = 0.0
                          # "This timer was placed here because the entire for loop should take approximatly 10s and this timer ensures it. In the next for loop iteration the currents are corrected, but since that is not part of this log entry, it is done after this long wait statement."
                          # "Pass the shift registers on."
                          # "The answer back from the PS is in the form x A. This A needs to be removed, otherwise the table formats wrong."
                          # "Request current CH3; write it to the file; put it on the current Z shift register"
                          n92 = call "Request current CH3 (SubVI).vi"() -> ("Request current CH3 / Z"=w361:string)  [unwired: 11 in]
                          n93 = VISA Write(VISA resource name=w360, write buffer=w361, error in (no error)=w359) -> (VISA resource name out=w371:refnum<visa-resource-name>, error out=w370:errorcluster)  [unwired: 1 out]
                          n94 = flat-sequence {
                            tunnel: w370 -> [w372]
                            tunnel: w371 -> [w373]
                            tunnel: [w373] -> w367
                            tunnel: u32 500 ("delay before read (ms) static") -> [w374]
                            tunnel: [w372] -> w366
                            frame #0 {
                              n95 = Wait (ms)(milliseconds to wait=w374) -> ()  [unwired: 1 out]
                            }
                          }
                          n96 = property class="Instr"(reference=w367, error in=w366) -> (reference out=w365:refnum<visa-resource-name>, error out=w363:errorcluster, "Serial Settings:Number of Bytes at Serial Port"=w364:u32)
                          n97 = VISA Read(VISA resource name=w365, byte count=w364, error in (no error)=w363) -> (VISA resource name out=w358:refnum<visa-resource-name>, read buffer=w368:string, error out=w357:errorcluster)  [unwired: 1 out]
                          n98 = Scan From String(format string="%fA", input string=w368) -> (output 1=w353:dbl)  [unwired: 3 in, 3 out]
                          n99 = Wait (ms)(milliseconds to wait=u32 3000) -> ()  [unwired: 1 out]
                          n100 = Number To Fractional String(number=w353) -> (F-format string=w356:string)  [unwired: 3 in]
                        }
                        frame 12 {
                          # "This is set here to avoid overloading the loop & power supply."
                          # "Pass the shift registers on."
                          # "In the first iteration of this while loop, current correction is executed with the connections slightly different, because I set hasn't updated correctly yet, which would  lead to errosrs.\nI is checked if the current flowing through the coils is what it should be , and corrected if necessary."
                          # "Send magnetic field Z to log file"
                          n101 = case shown="Default" w375 {
                            tunnel: w392 -> [w398 w436]
                            tunnel: w391 -> [_ w435]
                            tunnel: w390 -> [w399 w434]
                            tunnel: [w406 w433] -> w389
                            tunnel: [w400 w431] -> w388
                            tunnel: [w401 w430] -> w387
                            tunnel: w386 -> [w403 w429]
                            tunnel: w385 -> [w402 w428]
                            tunnel: w384 -> [w396 w426]
                            tunnel: w383 -> [_ w425]
                            tunnel: w382 -> [w397 w424]
                            tunnel: [w405 w423] -> w381
                            tunnel: w380 -> [w394 w421]
                            tunnel: w379 -> [w395 w420]
                            tunnel: w378 -> [_ w419]
                            tunnel: [w404 w418] -> w377
                            frame 0 {
                              n102 = call "Corrected current calculator (SubVI).vi"("Necessary current"=w397, "I_set old"=w397, "Actual current"=w396) -> ("I_set new"=w405:dbl)  [unwired: 8 in]
                              n103 = call "Corrected current calculator (SubVI).vi"("Necessary current"=w399, "I_set old"=w399, "Actual current"=w398) -> ("I_set new"=w406:dbl)  [unwired: 8 in]
                              n104 = call "Corrected current calculator (SubVI).vi"("Necessary current"=w395, "I_set old"=w395, "Actual current"=w394) -> ("I_set new"=w404:dbl)  [unwired: 8 in]
                              n105 = Number To Fractional String(number=w406) -> (F-format string=w413:string)  [unwired: 3 in]
                              n106 = Number To Fractional String(number=w405) -> (F-format string=w411:string)  [unwired: 3 in]
                              n107 = Number To Fractional String(number=w404) -> (F-format string=w410:string)  [unwired: 3 in]
                              n108 = call "Set I2 (SubVI).vi"("Current Y"=w411) -> ("String"=w408:string)  [unwired: 10 in]
                              n109 = call "Set I1 (SubVI).vi"("Current X"=w413) -> ("String instruction"=w407:string)  [unwired: 10 in]
                              n110 = call "Set I3 (SubVI).vi"("Current Z"=w410) -> ("String"=w409:string)  [unwired: 10 in]
                              n111 = Concatenate Strings(w407, w408, w409) -> (w412:string)
                              n112 = VISA Write(VISA resource name=w403, write buffer=w412, error in (no error)=w402) -> (VISA resource name out=w400:refnum<visa-resource-name>, error out=w401:errorcluster)  [unwired: 1 out]
                            }
                            frame Default {
                              # "Correct currents: calculate the new necessary current value; send the new current value to the power supply; place this newt I set on the while loop shift register."
                              n113 = call "Corrected current calculator (SubVI).vi"("Necessary current"=w424, "I_set old"=w425, "Actual current"=w426) -> ("I_set new"=w423:dbl)  [unwired: 8 in]
                              n114 = call "Corrected current calculator (SubVI).vi"("Necessary current"=w434, "I_set old"=w435, "Actual current"=w436) -> ("I_set new"=w433:dbl)  [unwired: 8 in]
                              n115 = call "Corrected current calculator (SubVI).vi"("Necessary current"=w420, "I_set old"=w419, "Actual current"=w421) -> ("I_set new"=w418:dbl)  [unwired: 8 in]
                              n116 = Number To Fractional String(number=w433) -> (F-format string=w432:string)  [unwired: 3 in]
                              n117 = Number To Fractional String(number=w423) -> (F-format string=w422:string)  [unwired: 3 in]
                              n118 = Number To Fractional String(number=w418) -> (F-format string=w417:string)  [unwired: 3 in]
                              n119 = call "Set I2 (SubVI).vi"("Current Y"=w422) -> ("String"=w415:string)  [unwired: 10 in]
                              n120 = call "Set I1 (SubVI).vi"("Current X"=w432) -> ("String instruction"=w414:string)  [unwired: 10 in]
                              n121 = call "Set I3 (SubVI).vi"("Current Z"=w417) -> ("String"=w416:string)  [unwired: 10 in]
                              n122 = Concatenate Strings(w414, w415, w416) -> (w427:string)
                              n123 = VISA Write(VISA resource name=w429, write buffer=w427, error in (no error)=w428) -> (VISA resource name out=w431:refnum<visa-resource-name>, error out=w430:errorcluster)  [unwired: 1 out]
                            }
                          }
                          n124 = call "Z Coil Current to Magnetic field (SubVI).vi"("Current Z"=w380) -> ("Magnetic field Z [µT]"=w393:string)  [unwired: 10 in]
                          n125 = Wait (ms)(milliseconds to wait=u32 1000) -> ()  [unwired: 1 out]
                        }
                      }
                      n126 = Wait (ms)(milliseconds to wait=u32 500) -> ()  [unwired: 1 out]
                    }
                    n127 = feedback-in #4(w129) -> ()
                    n128 = feedback-in #5(w134) -> ()
                    n129 = feedback-in #6(w132) -> ()
                    n130 = call-poly <vilib>:"Write Delimited Spreadsheet.vi"("file path (dialog if empty)"=w141, "1D data"=w142, "append to file? (new file:F)"=TRUE, "delimiter (\\t)"="," ("delimiter (\\t)")) -> ()  [unwired: 10 in, 2 out]
                  }
                  n131 = feedback-in #1(w98) -> ()
                  n132 = feedback-in #2(w97) -> ()
                  n133 = feedback-in #3(w95) -> ()
                }
              }
            }
          }
        }
      }
      frame "Static field" {
        n134 = case shown="True" "OK Button" {
          tunnel: w445 -> [w450 w462]
          tunnel: w441 -> [w449 w461]
          tunnel: [w448 w464] -> w444
          tunnel: [w447 w463] -> w443
          tunnel: "Magnetic field strength x [µT]" -> [_ w465]
          tunnel: "Magnetic field strength y [µT]" -> [_ _]
          tunnel: "file path static" -> [_ w468]
          tunnel: "Magnetic field strength z [µT]" -> [_ w467]
          tunnel: "Magnetic field strength y [µT]" -> [_ w466]
          frame False {
            # "If the stop button is pressed -> turn the channels off"
            n135 = local read "OFF"() -> (w446:bool)
            n136 = case shown="False" w446 {
              tunnel: w450 -> [w453 w460]
              tunnel: w449 -> [w452 w459]
              tunnel: [w455 w458] -> w448
              tunnel: [w454 w457] -> w447
              frame False {
                n137 = VISA Write(VISA resource name=w452, write buffer="0\n", error in (no error)=w453) -> (VISA resource name out=w454:refnum<visa-resource-name>, error out=w455:errorcluster)  [unwired: 1 out]
              }
              frame True {
                n138 = call "Turn channels off (subVI).vi"() -> ("String"=w456:string)  [unwired: 11 in]
                n139 = VISA Write(VISA resource name=w459, write buffer=w456, error in (no error)=w460) -> (VISA resource name out=w457:refnum<visa-resource-name>, error out=w458:errorcluster)  [unwired: 1 out]
              }
            }
          }
          frame True {
            # "Why this approach?\nFlat Sequence Structure ensures that headers are only written once at the start.\nCSV format is used because it’s simple, human-readable, and Excel-compatible.\nWhile Loop for data ensures real-time, continuous data logging."
            # "A flat sequence structure has been created here, to ensure a proper \"start\" to the file logging. \nFirst, the headers of each column aree initialised (of which there are 11). \nAfter that, the for loop (controlling the field sweep) starts executing."
            # "IF this mode is turned on:\nThe logging file is initialised. Then, the initial instructions are sent to the power supply: \n1. Set the initial values for the current\n2. Set the voltage limits\n3. Turn all the channels on\nAfter the initial currents are set, the script request the actual current from the power supply, reads it, compares it to the target value, and corrects it if necessary. \nThe current system state (which includes the iteration step, timestamp, voltage, current, and magnetic field strength for each coil) must be logged continuously at approximately 10-second intervals. Both the logging and feedback control processes run continuously after the new current values are sent, untill the stop button is pressed"
            n140 = flat-sequence {
              tunnel: w468 -> [w471]
              tunnel: [w470] -> w469
              tunnel: w461 -> [w506]
              tunnel: [w489] -> _
              tunnel: [w505] -> w463
              tunnel: w469 -> [w504]
              tunnel: w467 -> [w497]
              tunnel: w466 -> [w496]
              tunnel: w465 -> [w495]
              tunnel: [w490] -> w464
              tunnel: w462 -> [w489]
              frame #0 {
                # "Each iteration uses a Case Structure to determine which header to write.\nThese are constants and never change during execution."
                # "This formatting dictates that the file should be written to a csv comma delimited excell file."
                # "First, the headers of the file are initialised:\nEach iteration is a column:\n0. Iteration\n1. Set the time stamp\n2. Voltage X\n3. Current X\n4. Magnetic field X\n5. Voltage Y\n6. Current Y\n7. Magnetic field Y\n8. Voltage Z\n9. Current Z\n10. Magnetic field Z"
                n141 = for {
                  N: 11 -> [_]
                  tunnel: [w475] -> w473 mode=indexing
                  i -> [w476]
                  n142 = case shown="10" w476 {
                    tunnel: ["Iteration" "Time stamp" "Voltage X (V)" "Current X (A)" "Magnetic field X (uT)" "Voltage Y (V)" "Current Y (A)" "Magnetic field Y (uT)" "Voltage Z (V)" "Current Z (A)" "Magnetic field Z (uT)"] -> w475
                    frame 0, Default {
                    }
                    frame 1 {
                    }
                    frame 2 {
                    }
                    frame 3 {
                    }
                    frame 4 {
                    }
                    frame 5 {
                    }
                    frame 6 {
                    }
                    frame 7 {
                    }
                    frame 8 {
                    }
                    frame 9 {
                    }
                    frame 10 {
                    }
                  }
                }
                n143 = call-poly <vilib>:"Write Delimited Spreadsheet.vi"("file path (dialog if empty)"=w471, "1D data"=w473, "delimiter (\\t)"="," ("delimiter (\\t)")) -> ("new file path (Not A Path if cancelled)"=w470:path)  [unwired: 11 in, 1 out]
              }
              frame #1 {
                # "Necessary current Z"
                # "Necessary current Y"
                # "Necessary current X"
                # "The initial values of I_set are set to the first value sent to the power supply, namely the \"start values\"."
                # "I set_Z"
                # "I set_Y"
                # "I set_Y"
                # "I set_Z"
                # "I set_X"
                # "I set_X"
                n144 = call "Static field instruction generator (SubVI).vi"("Magnetic field strength z [µT]"=w497, "Magnetic field strength y [µT]"=w496, "Magnetic field strength x [µT]"=w495) -> ("Necessary current Y"=w492:dbl, "Necessary current X"=w493:dbl, "Necessary current Z"=w491:dbl, "String"=w494:string)  [unwired: 5 in]
                n145 = feedback #7(w493) -> (w503:dbl)
                n146 = feedback #8(w492) -> (w500:dbl)
                n147 = feedback #9(w491) -> (w498:dbl)
                n148 = while {
                  tunnel: w504 -> [w534]
                  tunnel: w506 -> [w531]
                  tunnel: w489 -> [w530]
                  tunnel: [w529] -> w490
                  tunnel: [w528] -> w505
                  tunnel: 0 -> [w521]
                  shift-right: [w520] -> w502
                  shift-left: w503 -> [w519]
                  tunnel: w494 -> [w518]
                  shift-right: [w517] -> w501
                  shift-left: w500 -> [w515]
                  shift-right: [w516] -> w499
                  shift-left: w498 -> [w514]
                  tunnel: w493 -> [w513]
                  tunnel: w492 -> [w512]
                  tunnel: w491 -> [w511]
                  i -> [w510]
                  stop <- "OFF" stop-if-true
                  w523 = 0.0
                  # "These shift registers \"remember\" the current actually flowing through the coils, which was obtained by querying the power supply."
                  # "Note that this while loop has three shift registers: I set_X, I set_Y, I set_Z.  These registers \"remember\" what current value has been set to the power supply. \nWhy? Well, when setting the maximal current value via the power supply the actual output current is consistently lower, generally by 0.1 to 0.5 mA.\nTo compensate this, it should request the actual current flowing through the coils from the power supply after the initial set command, read it, compare it to the target value, and correct it if necessary. To enable this process to execute continuously, these shift registers were added."
                  # "This while loop runs indefinitely until manually stopped by pressing the \"next iteration button\". \nLabVIEW writes the data using write to Spreadsheet File.vi (with comma delimiter), where the data is formatted as a 1D array per row.\nEvery loop iteration appends a new row to the file,, which takes about 11 seconds.  This data that it logs was obtained by communication with the power supply."
                  # "Necessary current Z"
                  # "Necessary current Y"
                  # "Necessary current X"
                  # "I set_Z"
                  # "I set_Y"
                  # "Iteration while loop"
                  # "Step of the sweep"
                  # "I set_X"
                  # "Actual current Z"
                  # "Actual current Y"
                  # "Actual current X"
                  # "Actual current Z"
                  # "Actual current Y"
                  # "Actual current X"
                  n149 = Greater Or Equal?(x=w510, y=1) -> (x >= y?=→"Current has stabilized":bool)
                  n150 = feedback #10(w523) -> (w536:dbl)
                  n151 = feedback #11(w523) -> (w526:dbl)
                  n152 = feedback #12(w523) -> (w524:dbl)
                  n153 = for {
                    N: 11 -> [_]
                    tunnel: [w560] -> w535 mode=indexing
                    shift-right: [w555] -> w522
                    shift-left: w536 -> [w562]
                    tunnel: "OFF" -> [w563]
                    tunnel: w531 -> [w559]
                    tunnel: w530 -> [w558]
                    tunnel: [w557] -> w529
                    tunnel: [w556] -> w528
                    shift-right: [w552] -> w527
                    shift-left: w526 -> [w554]
                    shift-right: [w551] -> w525
                    shift-left: w524 -> [w553]
                    tunnel: w510 -> [w550]
                    tunnel: w521 -> [w549]
                    tunnel: w519 -> [w548]
                    tunnel: [w547] -> w520
                    tunnel: w518 -> [w546]
                    tunnel: [w545] -> w517
                    tunnel: [w544] -> w516
                    tunnel: w515 -> [w543]
                    tunnel: w514 -> [w542]
                    tunnel: w513 -> [w541]
                    tunnel: w512 -> [w540]
                    tunnel: w511 -> [w539]
                    i -> [w561]
                    stop <- w563 stop-if-true
                    # "One row of data is logged per full finalisation of this for loop. Every iteration of this for loop is the value being added to that column of the row."
                    # "I set_Y"
                    # "I set_Z"
                    # "I set_X"
                    n154 = case shown="10" w561 {
                      tunnel: [w568 w591 w595 w622 w644 w654 w673 w696 w708 w731 w768] -> w560
                      tunnel: w559 -> [w571 w590 w610 w631 w646 w656 w680 w700 w710 w735 w761]
                      tunnel: w558 -> [w572 w589 w609 w632 w645 w655 w681 w701 w709 w734 w760]
                      tunnel: [w574 w590 w608 w634 w646 w650 w678 w700 w707 w733 w763] -> w556
                      tunnel: [w573 w589 w607 w633 w645 w649 w677 w701 w706 w732 w762] -> w557
                      tunnel: [w570 w588 w614 w623 w647 w653 w675 w699 w705 w730 w767] -> w555
                      tunnel: w562 -> [_ w588 w614 _ w647 w653 w675 w699 w705 w730 w767]
                      tunnel: w554 -> [_ w587 w598 w620 w643 w652 _ w697 w704 w729 w759]
                      tunnel: w553 -> [_ w586 w597 w619 w642 w651 w674 w698 w703 _ w755]
                      tunnel: [w570 w587 w598 w620 w643 w652 w676 w697 w704 w729 w759] -> w552
                      tunnel: [w570 w586 w597 w619 w642 w651 w674 w698 w703 w728 w755] -> w551
                      tunnel: w550 -> [w569 _ _ _ _ _ _ _ _ _ w750]
                      tunnel: w549 -> [w565 _ _ _ _ _ _ _ _ _ _]
                      tunnel: [w566 w585 w594 w618 w641 w648 w672 w695 w702 w727 w764] -> w547
                      tunnel: w548 -> [_ _ _ _ _ _ _ _ _ _ w766]
                      tunnel: w546 -> [w567 _ _ _ _ _ _ _ _ _ _]
                      tunnel: [w566 w585 w594 w618 w641 w648 w672 w695 w702 w727 w756] -> w545
                      tunnel: [w566 w585 w594 w618 w641 w648 w672 w695 w702 w727 w752] -> w544
                      tunnel: w543 -> [_ _ _ _ _ _ _ _ _ _ w758]
                      tunnel: w542 -> [_ _ _ _ _ _ _ _ _ _ w753]
                      tunnel: w541 -> [_ _ _ _ _ _ _ _ _ _ w765]
                      tunnel: w540 -> [_ _ _ _ _ _ _ _ _ _ w757]
                      tunnel: w539 -> [_ _ _ _ _ _ _ _ _ _ w754]
                      frame 0, Default {
                        w566 = 0.0
                        w570 = 0.0
                        # "Only the last value of I set values are sent through to the while loop shift registers (tunnel mode last value), so these values don't matter. \nThey are set to zero to make debugging easier).  The same thing is done in all other cases, except \"case 10\", which is the last iteration of this for loop."
                        # "The actual current flowing through the coils hasn't been queried yet,n so rthe \"actual current\" shift registers are set to zero (it could be set to any number, it was set to 0 to make debugging easier)."
                        # "If this is the first time this while loops has iterated, the start instructions are sent to the PS & the iteration number (of the large for loop, so which step of the sweep we are on) is sent to be logged in the table.\nElse, only the iteration number is sent to be logged in the table."
                        n155 = case shown="0" w569 {
                          tunnel: [w579 w584] -> w574
                          tunnel: [w578 w583] -> w573
                          tunnel: w572 -> [w577 w582]
                          tunnel: w571 -> [w576 w581]
                          tunnel: w567 -> [w575 _]
                          frame 0 {
                            n156 = VISA Write(VISA resource name=w576, write buffer=w575, error in (no error)=w577) -> (VISA resource name out=w579:refnum<visa-resource-name>, error out=w578:errorcluster)  [unwired: 1 out]
                          }
                          frame 1, Default {
                            n157 = VISA Write(VISA resource name=w581, write buffer="V4 0\n", error in (no error)=w582) -> (VISA resource name out=w584:refnum<visa-resource-name>, error out=w583:errorcluster)  [unwired: 1 out]
                          }
                        }
                        n158 = Wait (ms)(milliseconds to wait=u32 2000) -> ()  [unwired: 1 out]
                        n159 = Number To Decimal String(number=w565) -> (decimal integer string=w568:string)  [unwired: 1 in]
                      }
                      frame 1 {
                        w585 = 0.0
                        # "Nothing needs to be sent to the power supply."
                        # "Pass the shift registers on."
                        # "only send the time, not the date"
                        # "Send the time stamp to be logged"
                        n160 = Get Date/Time In Seconds() -> (seconds since 1Jan1904=w593:timestamp)
                        n161 = Format Date/Time String(time format string (%c)="%H:%M:%S", seconds (now)=w593) -> (date/time string=w591:string)  [unwired: 1 in]
                      }
                      frame 2 {
                        w594 = 0.0
                        # "Pass the shift registers on."
                        # "The answer back from the PS is in the form x V. This V needs to be removed, otherwise the table formats wrong."
                        # "Request voltage CH1 & write it to the file"
                        n162 = call "Request voltage CH1 (SubVI).vi"() -> ("Request voltage CH1 / X"=w600:string)  [unwired: 11 in]
                        n163 = VISA Write(VISA resource name=w610, write buffer=w600, error in (no error)=w609) -> (VISA resource name out=w613:refnum<visa-resource-name>, error out=w612:errorcluster)  [unwired: 1 out]
                        n164 = flat-sequence {
                          tunnel: w612 -> [w615]
                          tunnel: w613 -> [w616]
                          tunnel: [w616] -> w606
                          tunnel: u32 500 ("delay before read (ms) static") -> [w617]
                          tunnel: [w615] -> w605
                          frame #0 {
                            n165 = Wait (ms)(milliseconds to wait=w617) -> ()  [unwired: 1 out]
                          }
                        }
                        n166 = property class="Instr"(reference=w606, error in=w605) -> (reference out=w604:refnum<visa-resource-name>, error out=w603:errorcluster, "Serial Settings:Number of Bytes at Serial Port"=w602:u32)
                        n167 = VISA Read(VISA resource name=w604, byte count=w602, error in (no error)=w603) -> (VISA resource name out=w608:refnum<visa-resource-name>, read buffer=w599:string, error out=w607:errorcluster)  [unwired: 1 out]
                        n168 = Scan From String(format string="%fV", input string=w599) -> (output 1=w596:dbl)  [unwired: 3 in, 3 out]
                        n169 = Number To Fractional String(number=w596) -> (F-format string=w595:string)  [unwired: 3 in]
                      }
                      frame 3 {
                        w618 = 0.0
                        # "Pass the shift registers on."
                        # "The answer back from the PS is in the form x A. This A needs to be removed, otherwise the table formats wrong."
                        # "Request current CH1; write it to the file; put it on the current X shift register"
                        n170 = call "Request current CH1(SubVI).vi"() -> ("Request current CH1 / X"=w624:string)  [unwired: 11 in]
                        n171 = VISA Write(VISA resource name=w631, write buffer=w624, error in (no error)=w632) -> (VISA resource name out=w637:refnum<visa-resource-name>, error out=w636:errorcluster)  [unwired: 1 out]
                        n172 = flat-sequence {
                          tunnel: w636 -> [w638]
                          tunnel: w637 -> [w639]
                          tunnel: [w639] -> w629
                          tunnel: u32 500 ("delay before read (ms) static") -> [w640]
                          tunnel: [w638] -> w628
                          frame #0 {
                            n173 = Wait (ms)(milliseconds to wait=w640) -> ()  [unwired: 1 out]
                          }
                        }
                        n174 = property class="Instr"(reference=w629, error in=w628) -> (reference out=w627:refnum<visa-resource-name>, error out=w625:errorcluster, "Serial Settings:Number of Bytes at Serial Port"=w626:u32)
                        n175 = VISA Read(VISA resource name=w627, byte count=w626, error in (no error)=w625) -> (VISA resource name out=w634:refnum<visa-resource-name>, read buffer=w630:string, error out=w633:errorcluster)  [unwired: 1 out]
                        n176 = Scan From String(format string="%fA", input string=w630) -> (output 1=w623:dbl)  [unwired: 3 in, 3 out]
                        n177 = Number To Fractional String(number=w623) -> (F-format string=w622:string)  [unwired: 3 in]
                      }
                      frame 4 {
                        w641 = 0.0
                        # "Pass the shift registers on."
                        # "Send magnetic field X to log file"
                        n178 = call "X Coil Current to Magnetic field (SubVI).vi"("Current X"=w647) -> ("Magnetic field X [µT]"=w644:string)  [unwired: 10 in]
                      }
                      frame 5 {
                        w648 = 0.0
                        # "Pass the shift registers on."
                        # "The answer back from the PS is in the form x V. This V needs to be removed, otherwise the table formats wrong."
                        # "Request voltage CH2 & write it to the file"
                        n179 = call "Request voltage CH2 (SubVI).vi"() -> ("Request voltage CH2 / Y"=w657:string)  [unwired: 11 in]
                        n180 = VISA Write(VISA resource name=w656, write buffer=w657, error in (no error)=w655) -> (VISA resource name out=w668:refnum<visa-resource-name>, error out=w667:errorcluster)  [unwired: 1 out]
                        n181 = flat-sequence {
                          tunnel: w667 -> [w669]
                          tunnel: w668 -> [w670]
                          tunnel: [w670] -> w665
                          tunnel: u32 500 ("delay before read (ms) static") -> [w671]
                          tunnel: [w669] -> w664
                          frame #0 {
                            n182 = Wait (ms)(milliseconds to wait=w671) -> ()  [unwired: 1 out]
                          }
                        }
                        n183 = property class="Instr"(reference=w665, error in=w664) -> (reference out=w663:refnum<visa-resource-name>, error out=w662:errorcluster, "Serial Settings:Number of Bytes at Serial Port"=w661:u32)
                        n184 = VISA Read(VISA resource name=w663, byte count=w661, error in (no error)=w662) -> (VISA resource name out=w650:refnum<visa-resource-name>, read buffer=w659:string, error out=w649:errorcluster)  [unwired: 1 out]
                        n185 = Scan From String(format string="%fV", input string=w659) -> (output 1=w658:dbl)  [unwired: 3 in, 3 out]
                        n186 = Number To Fractional String(number=w658) -> (F-format string=w654:string)  [unwired: 3 in]
                      }
                      frame 6 {
                        w672 = 0.0
                        # "Pass the shift registers on."
                        # "The answer back from the PS is in the form x A. This A needs to be removed, otherwise the table formats wrong."
                        # "Request current CH2; write it to the file; put it on the current Y shift register"
                        n187 = call "Request current CH2 (SubVI).vi"() -> ("Request current CH2 / Y"=w679:string)  [unwired: 11 in]
                        n188 = VISA Write(VISA resource name=w680, write buffer=w679, error in (no error)=w681) -> (VISA resource name out=w691:refnum<visa-resource-name>, error out=w690:errorcluster)  [unwired: 1 out]
                        n189 = flat-sequence {
                          tunnel: w690 -> [w692]
                          tunnel: w691 -> [w693]
                          tunnel: [w693] -> w687
                          tunnel: u32 500 ("delay before read (ms) static") -> [w694]
                          tunnel: [w692] -> w686
                          frame #0 {
                            n190 = Wait (ms)(milliseconds to wait=w694) -> ()  [unwired: 1 out]
                          }
                        }
                        n191 = property class="Instr"(reference=w687, error in=w686) -> (reference out=w685:refnum<visa-resource-name>, error out=w683:errorcluster, "Serial Settings:Number of Bytes at Serial Port"=w684:u32)
                        n192 = VISA Read(VISA resource name=w685, byte count=w684, error in (no error)=w683) -> (VISA resource name out=w678:refnum<visa-resource-name>, read buffer=w688:string, error out=w677:errorcluster)  [unwired: 1 out]
                        n193 = Scan From String(format string="%fA", input string=w688) -> (output 1=w676:dbl)  [unwired: 3 in, 3 out]
                        n194 = Number To Fractional String(number=w676) -> (F-format string=w673:string)  [unwired: 3 in]
                      }
                      frame 7 {
                        w695 = 0.0
                        # "Pass the shift registers on."
                        # "Send magnetic field Y to log file"
                        n195 = call "Y Coil Current to Magnetic field (SubVI).vi"("Current Y"=w697) -> ("Magnetic field Y [µT]"=w696:string)  [unwired: 10 in]
                      }
                      frame 8 {
                        w702 = 0.0
                        # "Pass the shift registers on."
                        # "The answer back from the PS is in the form x V. This V needs to be removed, otherwise the table formats wrong."
                        # "Request voltage CH3 & write it to the file"
                        n196 = call "Request voltage CH3 (SubVI).vi"() -> ("Request voltage CH3 / Z"=w711:string)  [unwired: 11 in]
                        n197 = VISA Write(VISA resource name=w710, write buffer=w711, error in (no error)=w709) -> (VISA resource name out=w722:refnum<visa-resource-name>, error out=w721:errorcluster)  [unwired: 1 out]
                        n198 = flat-sequence {
                          tunnel: w721 -> [w723]
                          tunnel: w722 -> [w724]
                          tunnel: [w724] -> w719
                          tunnel: u32 500 ("delay before read (ms) static") -> [w725]
                          tunnel: [w723] -> w718
                          frame #0 {
                            n199 = Wait (ms)(milliseconds to wait=w725) -> ()  [unwired: 1 out]
                          }
                        }
                        n200 = property class="Instr"(reference=w719, error in=w718) -> (reference out=w717:refnum<visa-resource-name>, error out=w716:errorcluster, "Serial Settings:Number of Bytes at Serial Port"=w715:u32)
                        n201 = VISA Read(VISA resource name=w717, byte count=w715, error in (no error)=w716) -> (VISA resource name out=w707:refnum<visa-resource-name>, read buffer=w713:string, error out=w706:errorcluster)  [unwired: 1 out]
                        n202 = Scan From String(format string="%fV", input string=w713) -> (output 1=w712:dbl)  [unwired: 3 in, 3 out]
                        n203 = Number To Fractional String(number=w712) -> (F-format string=w708:string)  [unwired: 3 in]
                      }
                      frame 9 {
                        w727 = 0.0
                        # "Pass the shift registers on."
                        # "The answer back from the PS is in the form x A. This A needs to be removed, otherwise the table formats wrong."
                        # "Request current CH3; write it to the file; put it on the current Z shift register"
                        n204 = call "Request current CH3 (SubVI).vi"() -> ("Request current CH3 / Z"=w736:string)  [unwired: 11 in]
                        n205 = VISA Write(VISA resource name=w735, write buffer=w736, error in (no error)=w734) -> (VISA resource name out=w746:refnum<visa-resource-name>, error out=w745:errorcluster)  [unwired: 1 out]
                        n206 = flat-sequence {
                          tunnel: w745 -> [w747]
                          tunnel: w746 -> [w748]
                          tunnel: [w748] -> w742
                          tunnel: u32 500 ("delay before read (ms) static") -> [w749]
                          tunnel: [w747] -> w741
                          frame #0 {
                            n207 = Wait (ms)(milliseconds to wait=w749) -> ()  [unwired: 1 out]
                          }
                        }
                        n208 = property class="Instr"(reference=w742, error in=w741) -> (reference out=w740:refnum<visa-resource-name>, error out=w738:errorcluster, "Serial Settings:Number of Bytes at Serial Port"=w739:u32)
                        n209 = Wait (ms)(milliseconds to wait=u32 3000) -> ()  [unwired: 1 out]
                        n210 = VISA Read(VISA resource name=w740, byte count=w739, error in (no error)=w738) -> (VISA resource name out=w733:refnum<visa-resource-name>, read buffer=w743:string, error out=w732:errorcluster)  [unwired: 1 out]
                        n211 = Scan From String(format string="%fA", input string=w743) -> (output 1=w728:dbl)  [unwired: 3 in, 3 out]
                        n212 = Number To Fractional String(number=w728) -> (F-format string=w731:string)  [unwired: 3 in]
                      }
                      frame 10 {
                        # "Pass the shift registers on."
                        # "In the first iteration of this while loop, current correction is executed with the connections slightly different, because I set hasn't updated correctly yet, which would  lead to errosrs.\nI is checked if the current flowing through the coils is what it should be , and corrected if necessary."
                        # "Send magnetic field Z to log file"
                        n213 = case shown="Default" w750 {
                          tunnel: w767 -> [w774 w811]
                          tunnel: w766 -> [_ w810]
                          tunnel: w765 -> [w773 w809]
                          tunnel: [w781 w808] -> w764
                          tunnel: [w778 w806] -> w763
                          tunnel: [w777 w805] -> w762
                          tunnel: w761 -> [w775 w804]
                          tunnel: w760 -> [w776 w803]
                          tunnel: w759 -> [w772 w801]
                          tunnel: w758 -> [_ w800]
                          tunnel: w757 -> [w771 w799]
                          tunnel: [w780 w798] -> w756
                          tunnel: w755 -> [w770 w796]
                          tunnel: w754 -> [w769 w795]
                          tunnel: w753 -> [_ w794]
                          tunnel: [w779 w793] -> w752
                          frame 0 {
                            n214 = call "Corrected current calculator (SubVI).vi"("Necessary current"=w771, "I_set old"=w771, "Actual current"=w772) -> ("I_set new"=w780:dbl)  [unwired: 8 in]
                            n215 = call "Corrected current calculator (SubVI).vi"("Necessary current"=w773, "I_set old"=w773, "Actual current"=w774) -> ("I_set new"=w781:dbl)  [unwired: 8 in]
                            n216 = call "Corrected current calculator (SubVI).vi"("Necessary current"=w769, "I_set old"=w769, "Actual current"=w770) -> ("I_set new"=w779:dbl)  [unwired: 8 in]
                            n217 = Number To Fractional String(number=w781) -> (F-format string=w788:string)  [unwired: 3 in]
                            n218 = Number To Fractional String(number=w780) -> (F-format string=w786:string)  [unwired: 3 in]
                            n219 = Number To Fractional String(number=w779) -> (F-format string=w785:string)  [unwired: 3 in]
                            n220 = call "Set I2 (SubVI).vi"("Current Y"=w786) -> ("String"=w783:string)  [unwired: 10 in]
                            n221 = call "Set I1 (SubVI).vi"("Current X"=w788) -> ("String instruction"=w782:string)  [unwired: 10 in]
                            n222 = call "Set I3 (SubVI).vi"("Current Z"=w785) -> ("String"=w784:string)  [unwired: 10 in]
                            n223 = Concatenate Strings(w782, w783, w784) -> (w787:string)
                            n224 = VISA Write(VISA resource name=w775, write buffer=w787, error in (no error)=w776) -> (VISA resource name out=w778:refnum<visa-resource-name>, error out=w777:errorcluster)  [unwired: 1 out]
                          }
                          frame Default {
                            # "Correct currents: calculate the new necessary current value; send the new current value to the power supply; place this newt I set on the while loop shift register."
                            n225 = call "Corrected current calculator (SubVI).vi"("Necessary current"=w799, "I_set old"=w800, "Actual current"=w801) -> ("I_set new"=w798:dbl)  [unwired: 8 in]
                            n226 = call "Corrected current calculator (SubVI).vi"("Necessary current"=w809, "I_set old"=w810, "Actual current"=w811) -> ("I_set new"=w808:dbl)  [unwired: 8 in]
                            n227 = call "Corrected current calculator (SubVI).vi"("Necessary current"=w795, "I_set old"=w794, "Actual current"=w796) -> ("I_set new"=w793:dbl)  [unwired: 8 in]
                            n228 = Number To Fractional String(number=w808) -> (F-format string=w807:string)  [unwired: 3 in]
                            n229 = Number To Fractional String(number=w798) -> (F-format string=w797:string)  [unwired: 3 in]
                            n230 = Number To Fractional String(number=w793) -> (F-format string=w792:string)  [unwired: 3 in]
                            n231 = call "Set I2 (SubVI).vi"("Current Y"=w797) -> ("String"=w790:string)  [unwired: 10 in]
                            n232 = call "Set I1 (SubVI).vi"("Current X"=w807) -> ("String instruction"=w789:string)  [unwired: 10 in]
                            n233 = call "Set I3 (SubVI).vi"("Current Z"=w792) -> ("String"=w791:string)  [unwired: 10 in]
                            n234 = Concatenate Strings(w789, w790, w791) -> (w802:string)
                            n235 = VISA Write(VISA resource name=w804, write buffer=w802, error in (no error)=w803) -> (VISA resource name out=w806:refnum<visa-resource-name>, error out=w805:errorcluster)  [unwired: 1 out]
                          }
                        }
                        n236 = call "Z Coil Current to Magnetic field (SubVI).vi"("Current Z"=w755) -> ("Magnetic field Z [µT]"=w768:string)  [unwired: 10 in]
                        n237 = Wait (ms)(milliseconds to wait=u32 1000) -> ()  [unwired: 1 out]
                      }
                    }
                    n238 = Wait (ms)(milliseconds to wait=u32 500) -> ()  [unwired: 1 out]
                  }
                  n239 = feedback-in #10(w522) -> ()
                  n240 = feedback-in #11(w527) -> ()
                  n241 = feedback-in #12(w525) -> ()
                  n242 = call-poly <vilib>:"Write Delimited Spreadsheet.vi"("file path (dialog if empty)"=w534, "1D data"=w535, "append to file? (new file:F)"=TRUE, "delimiter (\\t)"="," ("delimiter (\\t)")) -> ()  [unwired: 10 in, 2 out]
                }
                n243 = feedback-in #7(w502) -> ()
                n244 = feedback-in #8(w501) -> ()
                n245 = feedback-in #9(w499) -> ()
              }
            }
          }
        }
      }
      frame "1D magnitude sweep" {
        n246 = case shown="True" "START" {
          tunnel: [w821 w823] -> w812
          tunnel: [w820 w825] -> w813
          tunnel: w815 -> [w818 w827]
          tunnel: w814 -> [w819 w826]
          frame False {
            n247 = VISA Write(VISA resource name=w818, write buffer="0\\n", error in (no error)=w819) -> (VISA resource name out=w821:refnum<visa-resource-name>, error out=w820:errorcluster)  [unwired: 1 out]
          }
          frame True {
            # "Why this approach?\nFlat Sequence Structure ensures that headers are only written once at the start.\nCSV format is used because it’s simple, human-readable, and Excel-compatible.\nWhile Loop for data ensures real-time, continuous data logging."
            # "A flat sequence structure has been created here, to ensure a proper \"start\" to the file logging. \nFirst, the headers of each column aree initialised (of which there are 11). \nAfter that, the for loop (controlling the field sweep) starts executing."
            n248 = flat-sequence {
              tunnel: "file path 1D" -> [w829]
              tunnel: [w828] -> w824
              tunnel: w827 -> [w846]
              tunnel: w826 -> [w845]
              tunnel: [w844] -> w823
              tunnel: [w843] -> w825
              tunnel: w824 -> [w842]
              frame #0 {
                # "Each iteration uses a Case Structure to determine which header to write.\nThese are constants and never change during execution."
                # "This formatting dictates that the file should be written to a csv comma delimited excell file."
                # "First, the headers of the file are initialised:\nEach iteration is a column:\n0. Iteration\n1. Set the time stamp\n2. Voltage X\n3. Current X\n4. Magnetic field X\n5. Voltage Y\n6. Current Y\n7. Magnetic field Y\n8. Voltage Z\n9. Current Z\n10. Magnetic field Z"
                n249 = for {
                  N: 6 -> [_]
                  tunnel: [w833] -> w831 mode=indexing
                  i -> [w834]
                  n250 = case shown="3" w834 {
                    tunnel: ["Iteration" "Time stamp" "Direction" "Voltage (V)" "Current (A)" "Magnetic field (uT)"] -> w833
                    frame 0, Default {
                    }
                    frame 1 {
                    }
                    frame 2 {
                    }
                    frame 3 {
                    }
                    frame 4 {
                    }
                    frame 5 {
                    }
                  }
                }
                n251 = call-poly <vilib>:"Write Delimited Spreadsheet.vi"("file path (dialog if empty)"=w829, "1D data"=w831, "delimiter (\\t)"="," ("delimiter (\\t)")) -> ("new file path (Not A Path if cancelled)"=w828:path)  [unwired: 11 in, 1 out]
              }
              frame #1 {
                # "# steps"
                # "This is the file path the values should be logged to."
                # "+2 is added to the total # of steps, as it also should include a step \"0\" (initialising all the terminals), and a final step that switches off all the channels."
                n252 = Increment(x="Number of steps") -> (x+1=w848:dbl)
                n253 = Increment(x=w848) -> (x+1=w847:dbl)
                n254 = for {
                  N: w847 -> [_]
                  tunnel: "Number of steps" -> [w856]
                  tunnel: w846 -> [w861]
                  tunnel: w845 -> [w860]
                  tunnel: [w859] -> w844
                  tunnel: [w858] -> w843
                  tunnel: w842 -> [w857]
                  i -> [w850]
                  stop <- FALSE stop-if-true
                  # "Direction field sweep"
                  # "All the necessary inputs are connected to the subVI here. The output string to be sent to the power supply is sent to the while loop"
                  # "Necessary current"
                  # "The initial values of I_set are set to the first value sent to the power supply, namely the \"start values\"."
                  # "This for loop works as follows: \nThe for loop consists of N+2 steps, and a new iteration is started when the \"next iteration button is pressed.\nWhen the N+2 steps have been executed, the loop is exited, and can be started again if wanted.\nEach loop iteration consists opf the same structure:\n1. The necesary instructions to be sent to the power supply for the new iteration are generated by the \"1D sweep iteration instruction generator\" SubVI. This has a range of user-defined values as inputs, and as output the generated instruction string to be sent to the power supply. It also has as outputs the magnetic field on each axis. These are connected to indicator to display the \"current state\" of the system, these values are then used in the following while loop.\n2. This while loop has two main functionalities: log the \"current state\" of the coils in an excell file & execute a feedback loop to ensure that the correct current is flowing through the coils, as this can drift over time. The workings of this while loop are described in the loop itself."
                  # "I set"
                  # "I set"
                  # "Required current in this iteration. \nUsed in the following while loop."
                  n255 = call "1D sweep iteration instruction generator (SubVI).vi"("Maximum value B [µT]"="Maximum value B [µT]", "Minimum value B [µT]"="Minimum value B [µT]", "Number of steps"=w856, "Current iteration"=w850, "Direction field sweep"="Direction field sweep") -> ("Current [µT]"=w852:dbl, "Magnetic field strength"=→"Magnetic field strength [µT]":dbl, "String"=w851:string)  [unwired: 4 in]
                  n256 = feedback #13(w852) -> (w863:dbl)
                  n257 = while {
                    tunnel: w857 -> [w883]
                    tunnel: w861 -> [w880]
                    tunnel: w860 -> [w879]
                    tunnel: [w878] -> w858
                    tunnel: [w877] -> w859
                    shift-right: [w874] -> w862
                    shift-left: w863 -> [w873]
                    tunnel: w851 -> [w872]
                    tunnel: w852 -> [w871]
                    tunnel: w850 -> [w867]
                    tunnel: "Direction field sweep" -> [w865]
                    i -> [w870]
                    stop <- w866 stop-if-true
                    # "These shift registers \"remember\" the current actually flowing through the coils, which was obtained by querying the power supply."
                    # "Note that this while loop has three shift registers: I set_X, I set_Y, I set_Z.  These registers \"remember\" what current value has been set to the power supply. \nWhy? Well, when setting the maximal current value via the power supply the actual output current is consistently lower, generally by 0.1 to 0.5 mA.\nTo compensate this, it should request the actual current flowing through the coils from the power supply after the initial set command, read it, compare it to the target value, and correct it if necessary. To enable this process to execute continuously, these shift registers were added."
                    # "This while loop runs indefinitely until manually stopped by pressing the \"next iteration button\". \nLabVIEW writes the data using write to Spreadsheet File.vi (with comma delimiter), where the data is formatted as a 1D array per row.\nEvery loop iteration appends a new row to the file,, which takes about 11 seconds.  This data that it logs was obtained by communication with the power supply."
                    # "Necessary current"
                    # "Iteration while loop"
                    # "Step of the sweep"
                    # "I set"
                    # "Actual current"
                    # "Actual current"
                    n258 = Greater Or Equal?(x=w870, y=1) -> (x >= y?=→"Current has stabilized":bool)
                    n259 = feedback #14(0.0) -> (w885:dbl)
                    n260 = for {
                      N: 6 -> [_]
                      tunnel: [w901] -> w884 mode=indexing
                      shift-right: [w896] -> w875
                      shift-left: w885 -> [w903]
                      tunnel: w880 -> [w900]
                      tunnel: w879 -> [w899]
                      tunnel: [w898] -> w878
                      tunnel: [w897] -> w877
                      tunnel: w870 -> [w895]
                      tunnel: w867 -> [w894]
                      tunnel: w873 -> [w893]
                      tunnel: [w892] -> w874
                      tunnel: w872 -> [w891]
                      tunnel: w871 -> [w890]
                      tunnel: ["Next iteration 2"] -> w866
                      tunnel: w865 -> [w887]
                      i -> [w902]
                      stop <- "Next iteration 2" stop-if-true
                      # "One row of data is logged per full finalisation of this for loop. Every iteration of this for loop is the value being added to that column of the row."
                      # "I set"
                      n261 = case shown="0, Default" w902 {
                        tunnel: [w908 w929 w934 w944 w971 w1002] -> w901
                        tunnel: w900 -> [w911 w928 w932 w956 w979 w996]
                        tunnel: w899 -> [w912 w927 w933 w955 w980 w995]
                        tunnel: [w914 w928 w932 w954 w982 w993] -> w897
                        tunnel: [w913 w927 w933 w953 w981 w992] -> w898
                        tunnel: [0.0 w926 w937 w960 w972 w1001] -> w896
                        tunnel: w903 -> [_ w926 w937 w960 _ w1001]
                        tunnel: w895 -> [w909 _ _ _ _ w997]
                        tunnel: w894 -> [w905 _ _ _ _ _]
                        tunnel: [0.0 0.0 0.0 0.0 0.0 w994] -> w892
                        tunnel: w893 -> [_ _ _ _ _ w1000]
                        tunnel: w891 -> [w907 _ _ _ _ _]
                        tunnel: w890 -> [_ _ _ _ _ w999]
                        tunnel: w887 -> [_ _ w935 w942 w968 w998]
                        frame 0, Default {
                          # "This timer is placed here so the power supply has enough time to execute all the instructions sent in the first step"
                          # "Only the last value of I set values are sent through to the while loop shift registers (tunnel mode last value), so these values don't matter. \nThey are set to zero to make debugging easier).  The same thing is done in all other cases, except \"case 10\", which is the last iteration of this for loop."
                          # "The actual current flowing through the coils hasn't been queried yet,n so rthe \"actual current\" shift registers are set to zero (it could be set to any number, it was set to 0 to make debugging easier)."
                          # "If this is the first time this while loops has iterated, the start instructions are sent to the PS & the iteration number (of the large for loop, so which step of the sweep we are on) is sent to be logged in the table.\nElse, only the iteration number is sent to be logged in the table."
                          n262 = case shown="0" w909 {
                            tunnel: [w919 w924] -> w914
                            tunnel: [w918 w923] -> w913
                            tunnel: w912 -> [w917 w922]
                            tunnel: w911 -> [w916 w921]
                            tunnel: w907 -> [w915 _]
                            frame 0 {
                              n263 = VISA Write(VISA resource name=w916, write buffer=w915, error in (no error)=w917) -> (VISA resource name out=w919:refnum<visa-resource-name>, error out=w918:errorcluster)  [unwired: 1 out]
                            }
                            frame 1, Default {
                              n264 = VISA Write(VISA resource name=w921, write buffer="V4 0\n", error in (no error)=w922) -> (VISA resource name out=w924:refnum<visa-resource-name>, error out=w923:errorcluster)  [unwired: 1 out]
                            }
                          }
                          n265 = Wait (ms)(milliseconds to wait=u32 4000) -> ()  [unwired: 1 out]
                          n266 = Number To Decimal String(number=w905) -> (decimal integer string=w908:string)  [unwired: 1 in]
                        }
                        frame 1 {
                          # "Nothing needs to be sent to the power supply."
                          # "Pass the shift registers on."
                          # "only send the time, not the date"
                          # "Send the time stamp to be logged"
                          n267 = Get Date/Time In Seconds() -> (seconds since 1Jan1904=w931:timestamp)
                          n268 = Format Date/Time String(time format string (%c)="%H:%M:%S", seconds (now)=w931) -> (date/time string=w929:string)  [unwired: 1 in]
                        }
                        frame 2 {
                          # "Pass the shift registers on."
                          # "Send the direction to be logged"
                          n269 = case shown="\"z\"" w935 {
                            tunnel: ["X" "Y" "Z"] -> w934
                            frame "x", Default {
                            }
                            frame "y" {
                            }
                            frame "z" {
                            }
                          }
                        }
                        frame 3 {
                          # "Pass the shift registers on."
                          # "The answer back from the PS is in the form x V. This V needs to be removed, otherwise the table formats wrong."
                          # "Request voltage of specified CH & write it to the file"
                          n270 = case shown="\"y\"" w942 {
                            tunnel: [w961 w962 w963] -> w941
                            frame "x", Default {
                              n271 = call "Request voltage CH1 (SubVI).vi"() -> ("Request voltage CH1 / X"=w961:string)  [unwired: 11 in]
                            }
                            frame "y" {
                              n272 = call "Request voltage CH2 (SubVI).vi"() -> ("Request voltage CH2 / Y"=w962:string)  [unwired: 11 in]
                            }
                            frame "z" {
                              n273 = call "Request voltage CH3 (SubVI).vi"() -> ("Request voltage CH3 / Z"=w963:string)  [unwired: 11 in]
                            }
                          }
                          n274 = VISA Write(VISA resource name=w956, write buffer=w941, error in (no error)=w955) -> (VISA resource name out=w959:refnum<visa-resource-name>, error out=w958:errorcluster)  [unwired: 1 out]
                          n275 = flat-sequence {
                            tunnel: w958 -> [w964]
                            tunnel: w959 -> [w965]
                            tunnel: [w965] -> w952
                            tunnel: u32 500 ("delay before read (ms) static") -> [w966]
                            tunnel: [w964] -> w951
                            frame #0 {
                              n276 = Wait (ms)(milliseconds to wait=w966) -> ()  [unwired: 1 out]
                            }
                          }
                          n277 = property class="Instr"(reference=w952, error in=w951) -> (reference out=w950:refnum<visa-resource-name>, error out=w949:errorcluster, "Serial Settings:Number of Bytes at Serial Port"=w948:u32)
                          n278 = VISA Read(VISA resource name=w950, byte count=w948, error in (no error)=w949) -> (VISA resource name out=w954:refnum<visa-resource-name>, read buffer=w946:string, error out=w953:errorcluster)  [unwired: 1 out]
                          n279 = Scan From String(format string="%fV", input string=w946) -> (output 1=w945:dbl)  [unwired: 3 in, 3 out]
                          n280 = Number To Fractional String(number=w945) -> (F-format string=w944:string)  [unwired: 3 in]
                        }
                        frame 4 {
                          # "Pass the shift registers on."
                          # "The answer back from the PS is in the form x A. This A needs to be removed, otherwise the table formats wrong."
                          # "Request current specified CH; write it to the file; put it on the current shift register"
                          n281 = case shown="\"z\"" w968 {
                            tunnel: [w986 w987 w988] -> w967
                            frame "x", Default {
                              n282 = call "Request current CH1(SubVI).vi"() -> ("Request current CH1 / X"=w986:string)  [unwired: 11 in]
                            }
                            frame "y" {
                              n283 = call "Request current CH2 (SubVI).vi"() -> ("Request current CH2 / Y"=w987:string)  [unwired: 11 in]
                            }
                            frame "z" {
                              n284 = call "Request current CH3 (SubVI).vi"() -> ("Request current CH3 / Z"=w988:string)  [unwired: 11 in]
                            }
                          }
                          n285 = VISA Write(VISA resource name=w979, write buffer=w967, error in (no error)=w980) -> (VISA resource name out=w985:refnum<visa-resource-name>, error out=w984:errorcluster)  [unwired: 1 out]
                          n286 = flat-sequence {
                            tunnel: w984 -> [w989]
                            tunnel: w985 -> [w990]
                            tunnel: [w990] -> w977
                            tunnel: u32 500 ("delay before read (ms) static") -> [w991]
                            tunnel: [w989] -> w976
                            frame #0 {
                              n287 = Wait (ms)(milliseconds to wait=w991) -> ()  [unwired: 1 out]
                            }
                          }
                          n288 = property class="Instr"(reference=w977, error in=w976) -> (reference out=w975:refnum<visa-resource-name>, error out=w973:errorcluster, "Serial Settings:Number of Bytes at Serial Port"=w974:u32)
                          n289 = VISA Read(VISA resource name=w975, byte count=w974, error in (no error)=w973) -> (VISA resource name out=w982:refnum<visa-resource-name>, read buffer=w978:string, error out=w981:errorcluster)  [unwired: 1 out]
                          n290 = Scan From String(format string="%fA", input string=w978) -> (output 1=w972:dbl)  [unwired: 3 in, 3 out]
                          n291 = Number To Fractional String(number=w972) -> (F-format string=w971:string)  [unwired: 3 in]
                        }
                        frame 5 {
                          # "This is set here to avoid overloading the loop & power supply."
                          # "Pass the shift registers on."
                          # "In the first iteration of this while loop, current correction is executed with the connections slightly different, because I set hasn't updated correctly yet, which would  lead to errosrs.\nI is checked if the current flowing through the coils is what it should be , and corrected if necessary."
                          # "Send magnetic field specified CH to log file"
                          n292 = case shown="0" w997 {
                            tunnel: [w1009 w1030] -> w994
                            tunnel: [w1011 w1029] -> w993
                            tunnel: [w1010 w1028] -> w992
                            tunnel: w996 -> [w1013 w1021]
                            tunnel: w995 -> [w1012 w1020]
                            tunnel: w1001 -> [w1007 w1027]
                            tunnel: w1000 -> [_ w1026]
                            tunnel: w999 -> [w1006 w1025]
                            tunnel: w998 -> [w1004 w1024]
                            frame 0 {
                              n293 = call "Corrected current calculator (SubVI).vi"("Necessary current"=w1006, "I_set old"=w1006, "Actual current"=w1007) -> ("I_set new"=w1009:dbl)  [unwired: 8 in]
                              n294 = Number To Fractional String(number=w1009) -> (F-format string=w1008:string)  [unwired: 3 in]
                              n295 = case shown="\"z\"" w1004 {
                                tunnel: w1008 -> [w1015 w1017 w1019]
                                tunnel: [w1014 w1016 w1018] -> w1005
                                frame "x", Default {
                                n296 = call "Set I1 (SubVI).vi"("Current X"=w1015) -> ("String instruction"=w1014:string)  [unwired: 10 in]
                                }
                                frame "y" {
                                n297 = call "Set I2 (SubVI).vi"("Current Y"=w1017) -> ("String"=w1016:string)  [unwired: 10 in]
                                }
                                frame "z" {
                                n298 = call "Set I3 (SubVI).vi"("Current Z"=w1019) -> ("String"=w1018:string)  [unwired: 10 in]
                                }
                              }
                              n299 = VISA Write(VISA resource name=w1013, write buffer=w1005, error in (no error)=w1012) -> (VISA resource name out=w1011:refnum<visa-resource-name>, error out=w1010:errorcluster)  [unwired: 1 out]
                            }
                            frame Default {
                              # "Correct currents: calculate the new necessary current value; send the new current value to the power supply; place this newt I set on the while loop shift register."
                              n300 = call "Corrected current calculator (SubVI).vi"("Necessary current"=w1025, "I_set old"=w1026, "Actual current"=w1027) -> ("I_set new"=w1030:dbl)  [unwired: 8 in]
                              n301 = Number To Fractional String(number=w1030) -> (F-format string=w1023:string)  [unwired: 3 in]
                              n302 = case shown="\"z\"" w1024 {
                                tunnel: w1023 -> [w1032 w1034 w1036]
                                tunnel: [w1031 w1033 w1035] -> w1022
                                frame "x", Default {
                                n303 = call "Set I1 (SubVI).vi"("Current X"=w1032) -> ("String instruction"=w1031:string)  [unwired: 10 in]
                                }
                                frame "y" {
                                n304 = call "Set I2 (SubVI).vi"("Current Y"=w1034) -> ("String"=w1033:string)  [unwired: 10 in]
                                }
                                frame "z" {
                                n305 = call "Set I3 (SubVI).vi"("Current Z"=w1036) -> ("String"=w1035:string)  [unwired: 10 in]
                                }
                              }
                              n306 = VISA Write(VISA resource name=w1021, write buffer=w1022, error in (no error)=w1020) -> (VISA resource name out=w1029:refnum<visa-resource-name>, error out=w1028:errorcluster)  [unwired: 1 out]
                            }
                          }
                          n307 = case shown="\"y\"" w998 {
                            tunnel: w1001 -> [w1038 w1040 w1042]
                            tunnel: [w1037 w1039 w1041] -> w1002
                            frame "x", Default {
                              n308 = call "X Coil Current to Magnetic field (SubVI).vi"("Current X"=w1038) -> ("Magnetic field X [µT]"=w1037:string)  [unwired: 10 in]
                            }
                            frame "y" {
                              n309 = call "Y Coil Current to Magnetic field (SubVI).vi"("Current Y"=w1040) -> ("Magnetic field Y [µT]"=w1039:string)  [unwired: 10 in]
                            }
                            frame "z" {
                              n310 = call "Z Coil Current to Magnetic field (SubVI).vi"("Current Z"=w1042) -> ("Magnetic field Z [µT]"=w1041:string)  [unwired: 10 in]
                            }
                          }
                          n311 = Wait (ms)(milliseconds to wait=u32 1000) -> ()  [unwired: 1 out]
                        }
                      }
                      n312 = Wait (ms)(milliseconds to wait=u32 500) -> ()  [unwired: 1 out]
                    }
                    n313 = feedback-in #14(w875) -> ()
                    n314 = call-poly <vilib>:"Write Delimited Spreadsheet.vi"("file path (dialog if empty)"=w883, "1D data"=w884, "append to file? (new file:F)"=TRUE, "delimiter (\\t)"="," ("delimiter (\\t)")) -> ()  [unwired: 10 in, 2 out]
                  }
                  n315 = feedback-in #13(w862) -> ()
                }
              }
            }
          }
        }
      }
    }
    n316 = VISA Close(VISA resource name=w7, error in (no error)=w6) -> (error out=w14:errorcluster)
    n317 = call <vilib>:"Simple Error Handler.vi"("error in (no error)"=w14) -> ()  [unwired: 1 in, 8 out]
  }
